vi "CRYGet Window Title Message.vi"(9 "Tooltip No":i32, 10 "No":i32, 11 "Kind":string) -> (0 "Control Label Off":string[](array[string]), 1 "Control Label On":string[](array[string]), 2 "Unicode String":string, 3 "Multibyte String":string, 4 "Control Name":string[](array[string]), 6 "Tip Strip":string[](array[string]))   [LabVIEW 2013]
uses:
  CRYMainGlobal.vi
panel:
  # "Get Window Title Message."
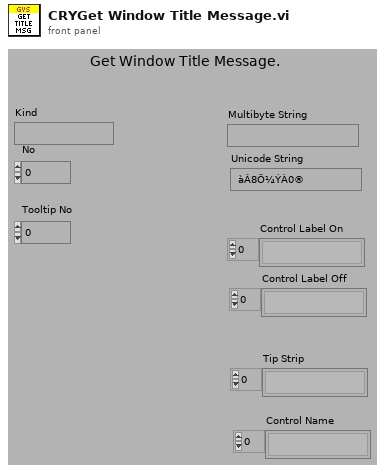
[diagram p1: front panel]
types:
  T1 = enum32{"English", "Chinese", "Korean", "Japanese", "Russian", "Chinese traditional"}
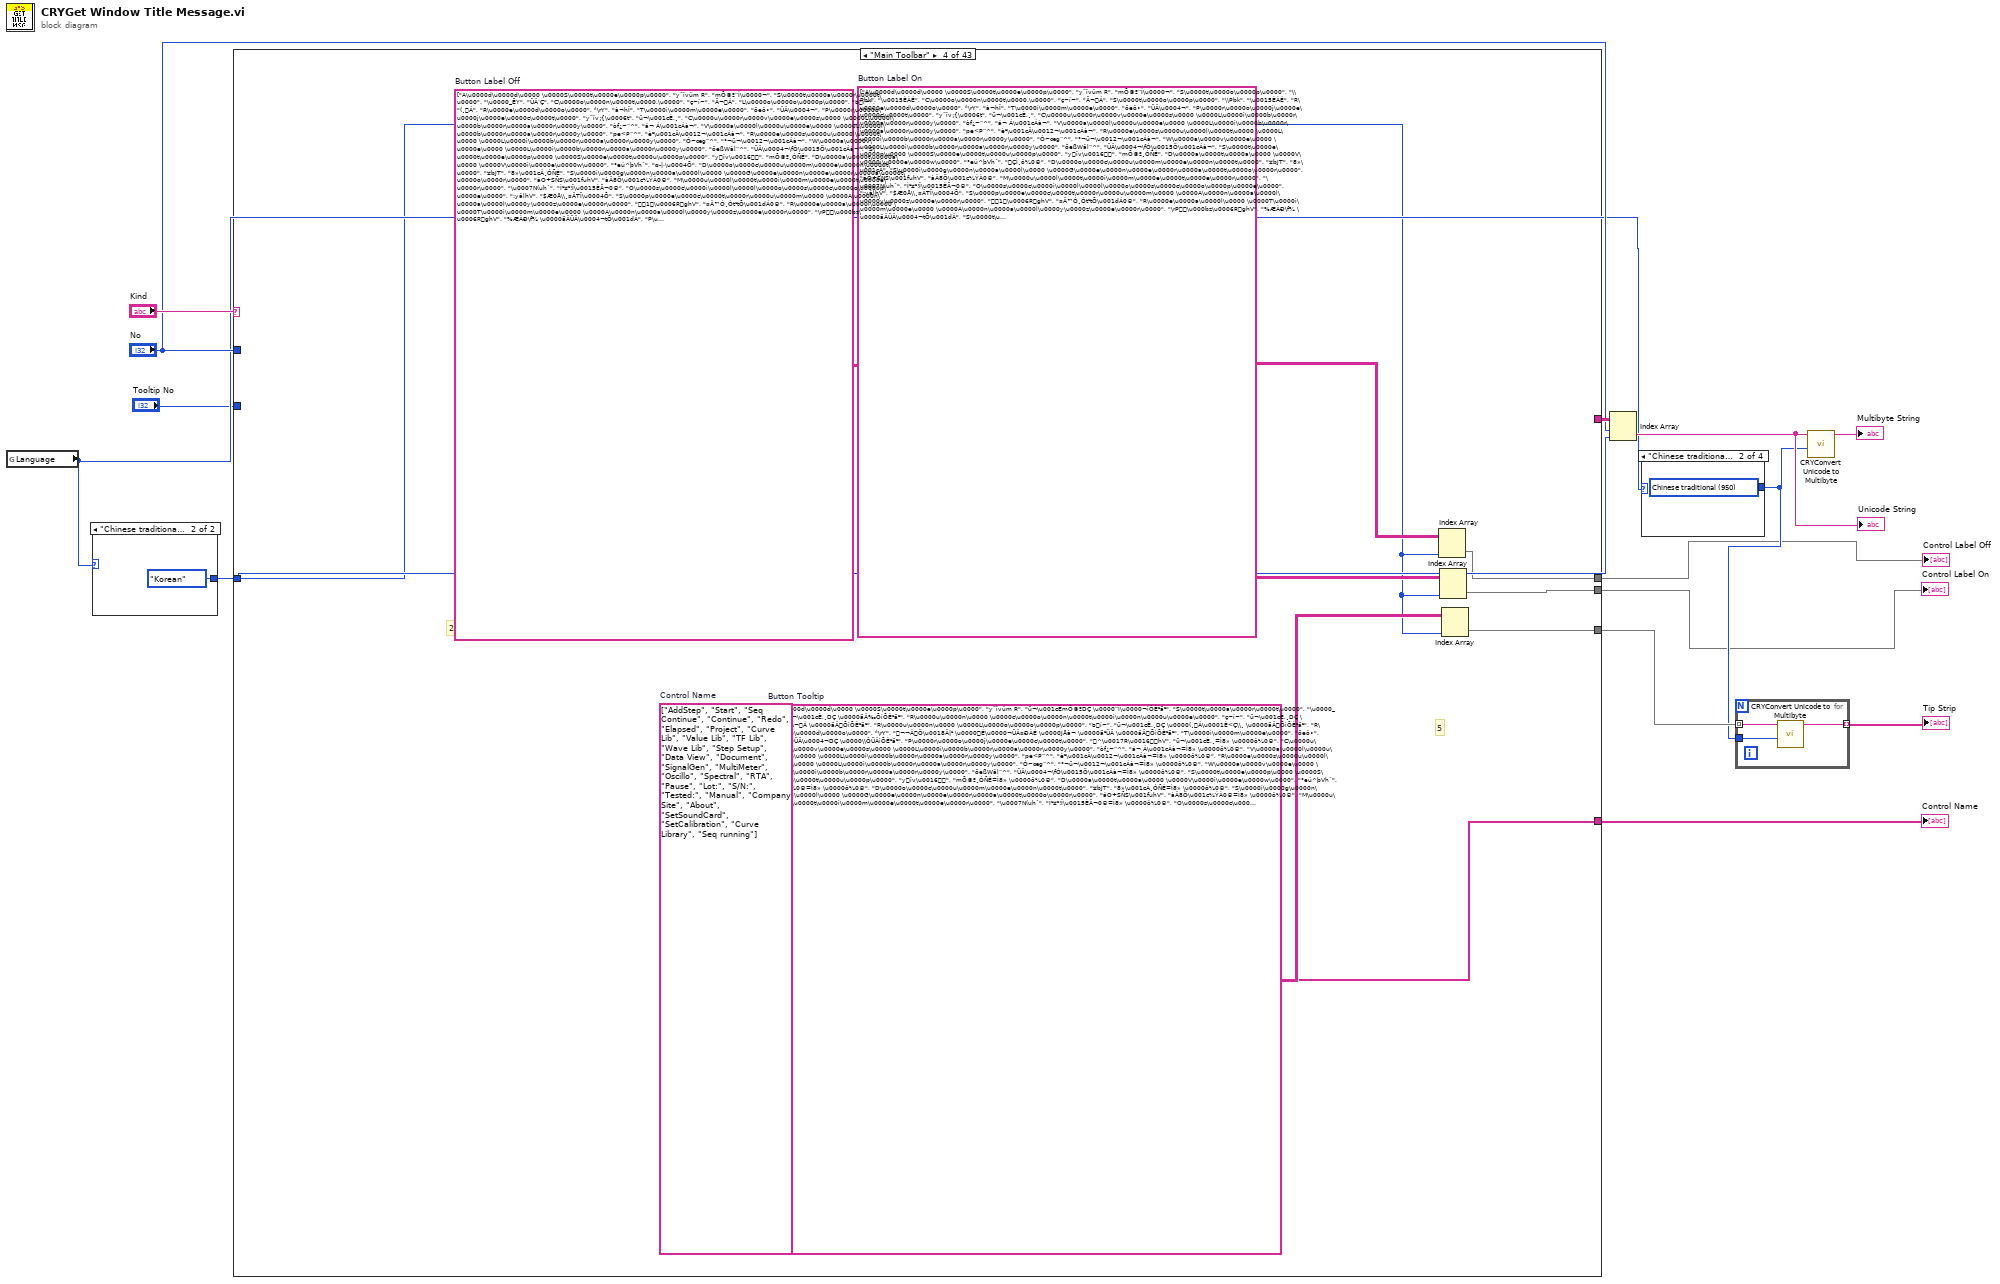
[diagram p0: block diagram]
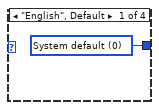
[diagram p3: hidden frame]
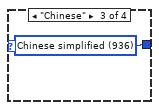
[diagram p4: hidden frame]
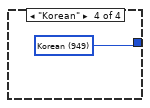
[diagram p5: hidden frame]
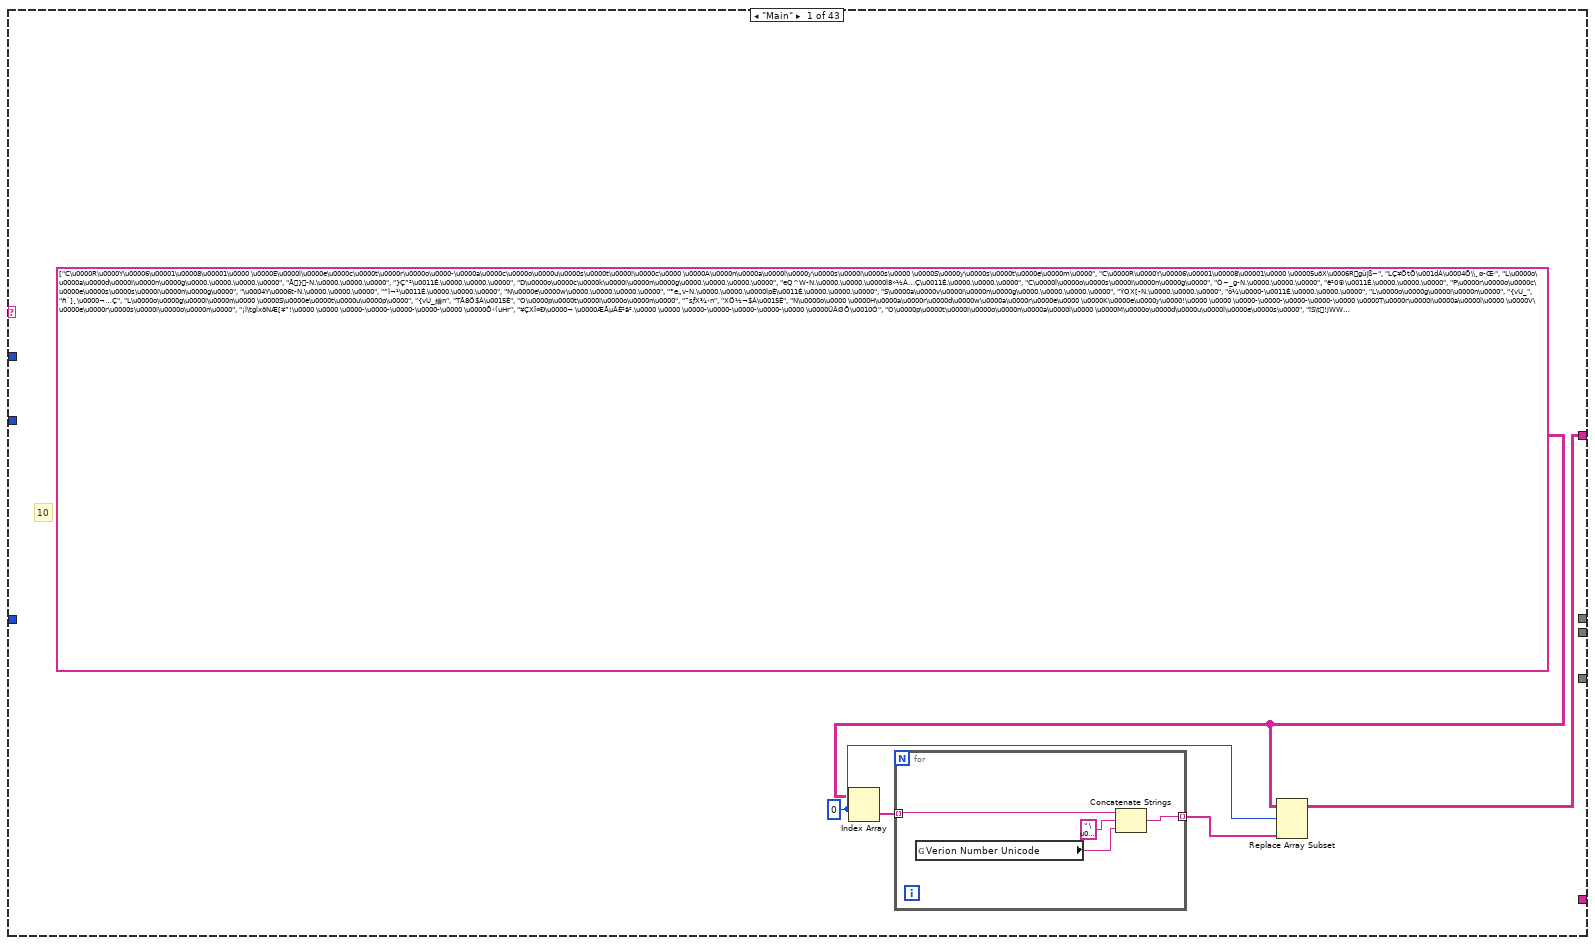
[diagram p6: hidden frame]
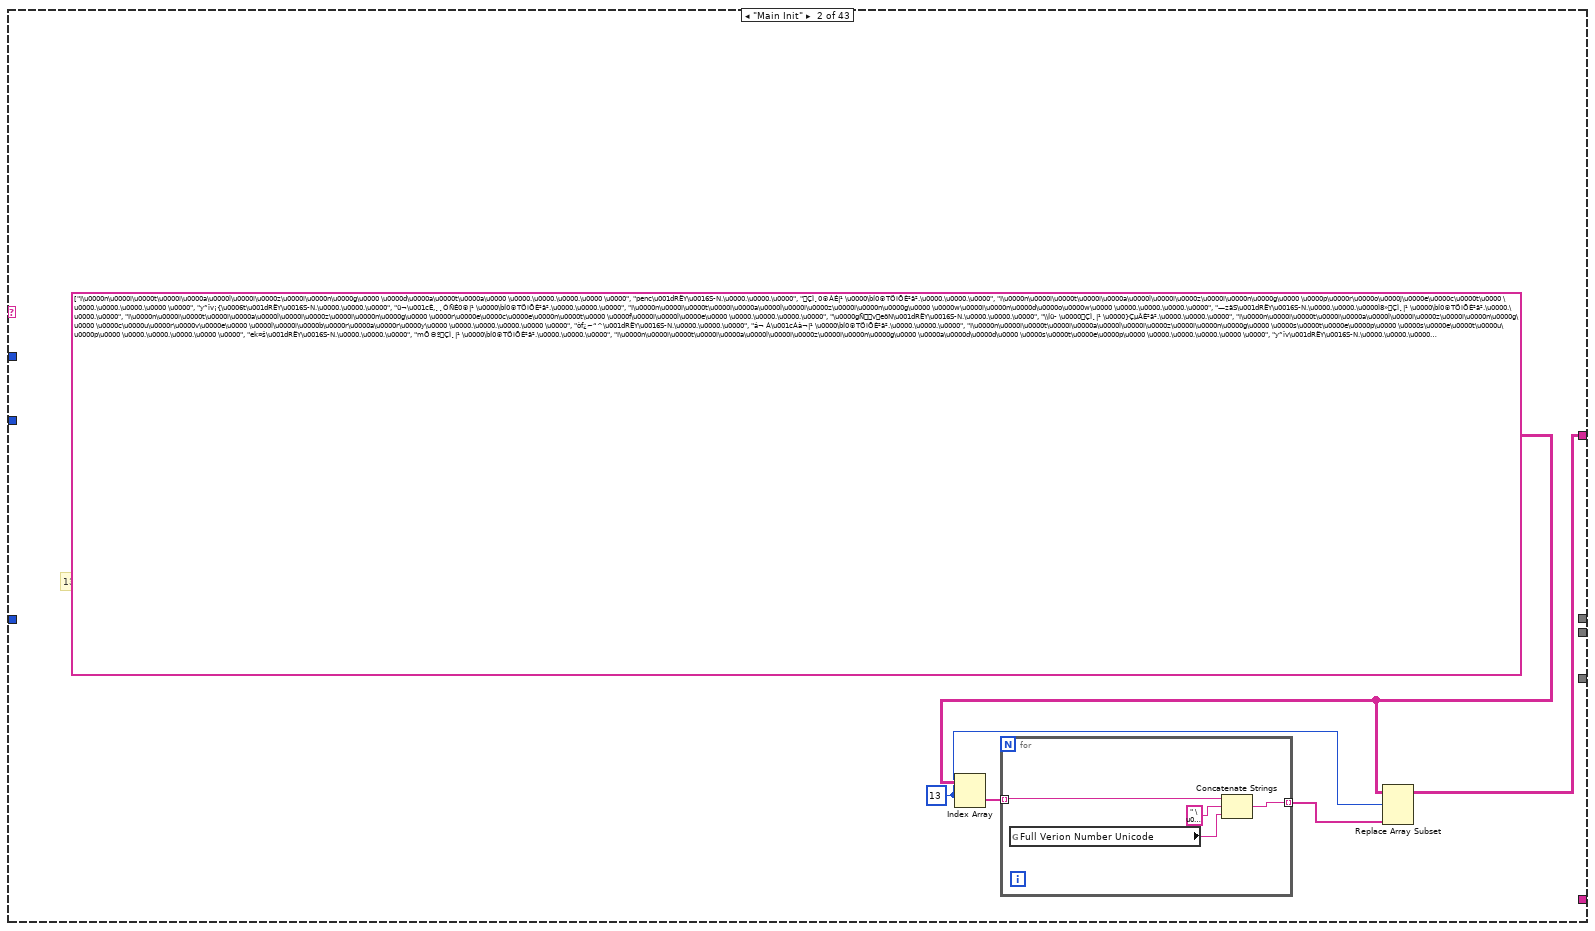
[diagram p7: hidden frame]
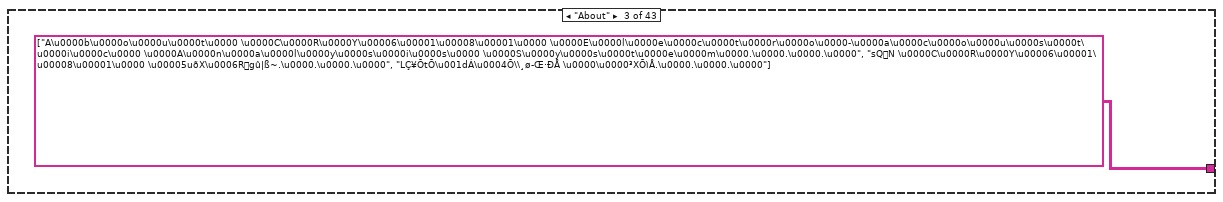
[diagram p8: hidden frame]
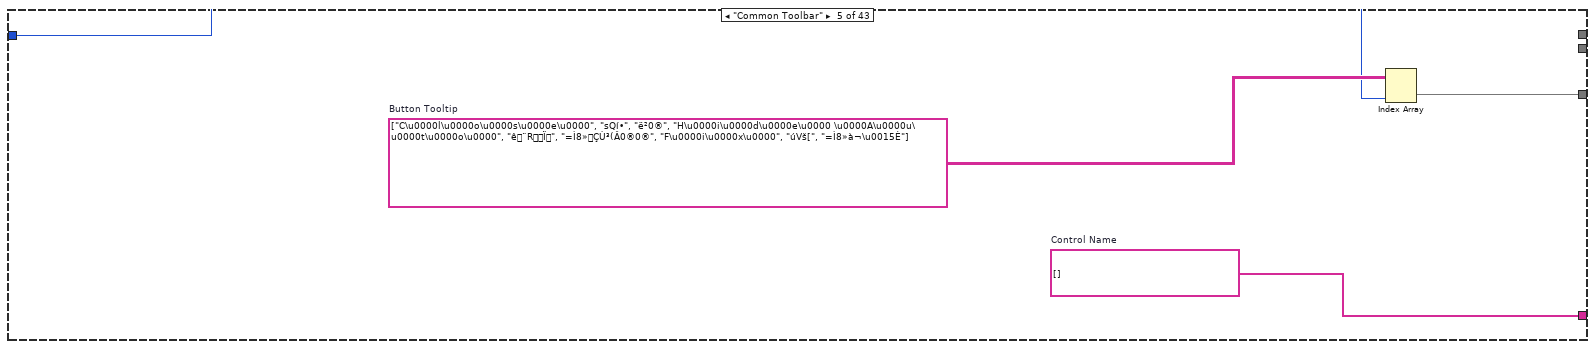
[diagram p9: hidden frame]
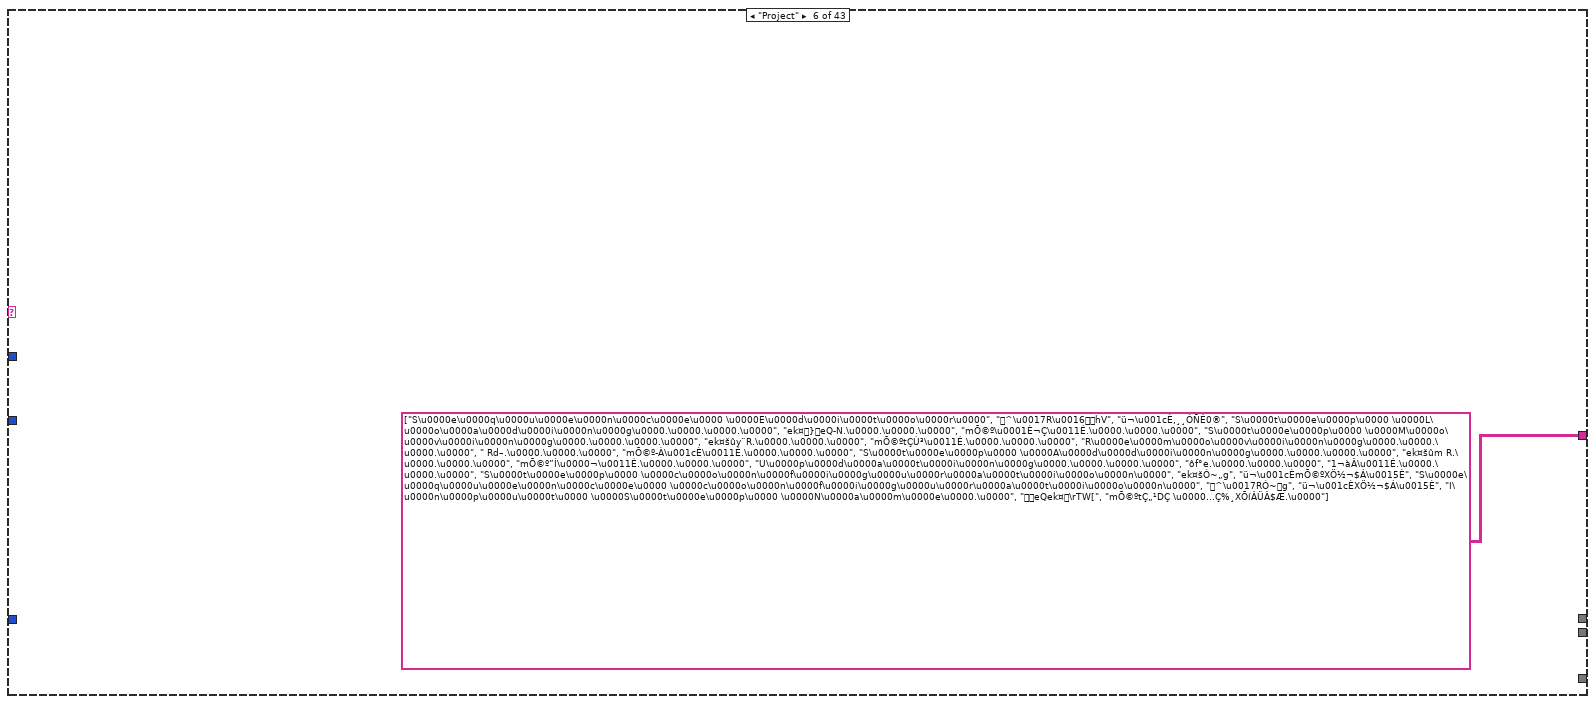
[diagram p10: hidden frame]
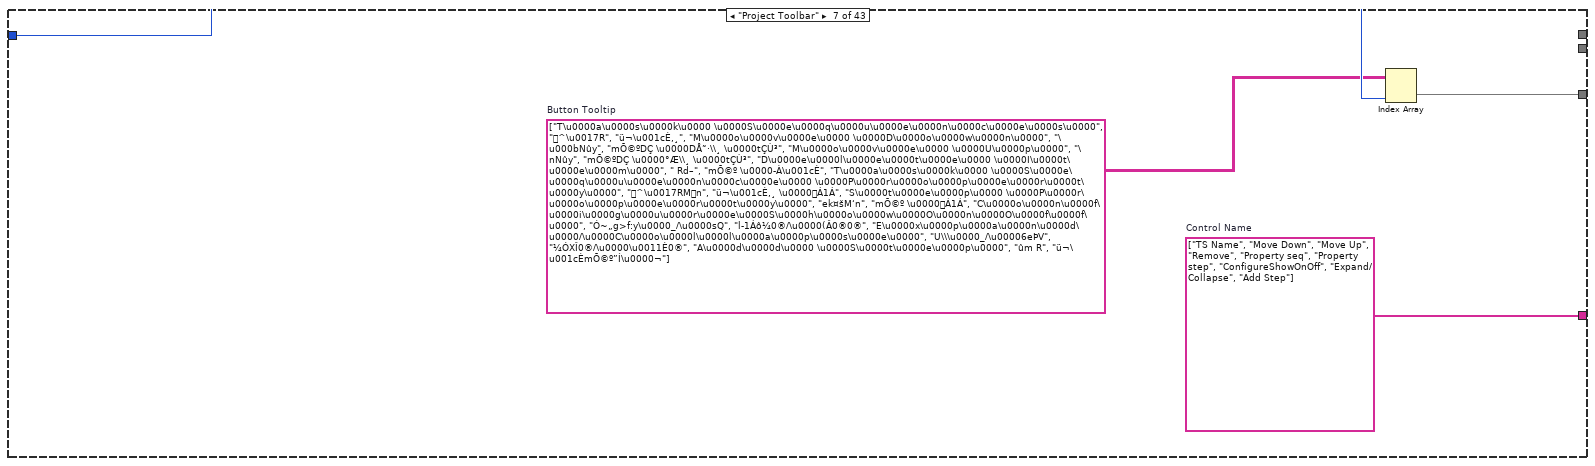
[diagram p11: hidden frame]
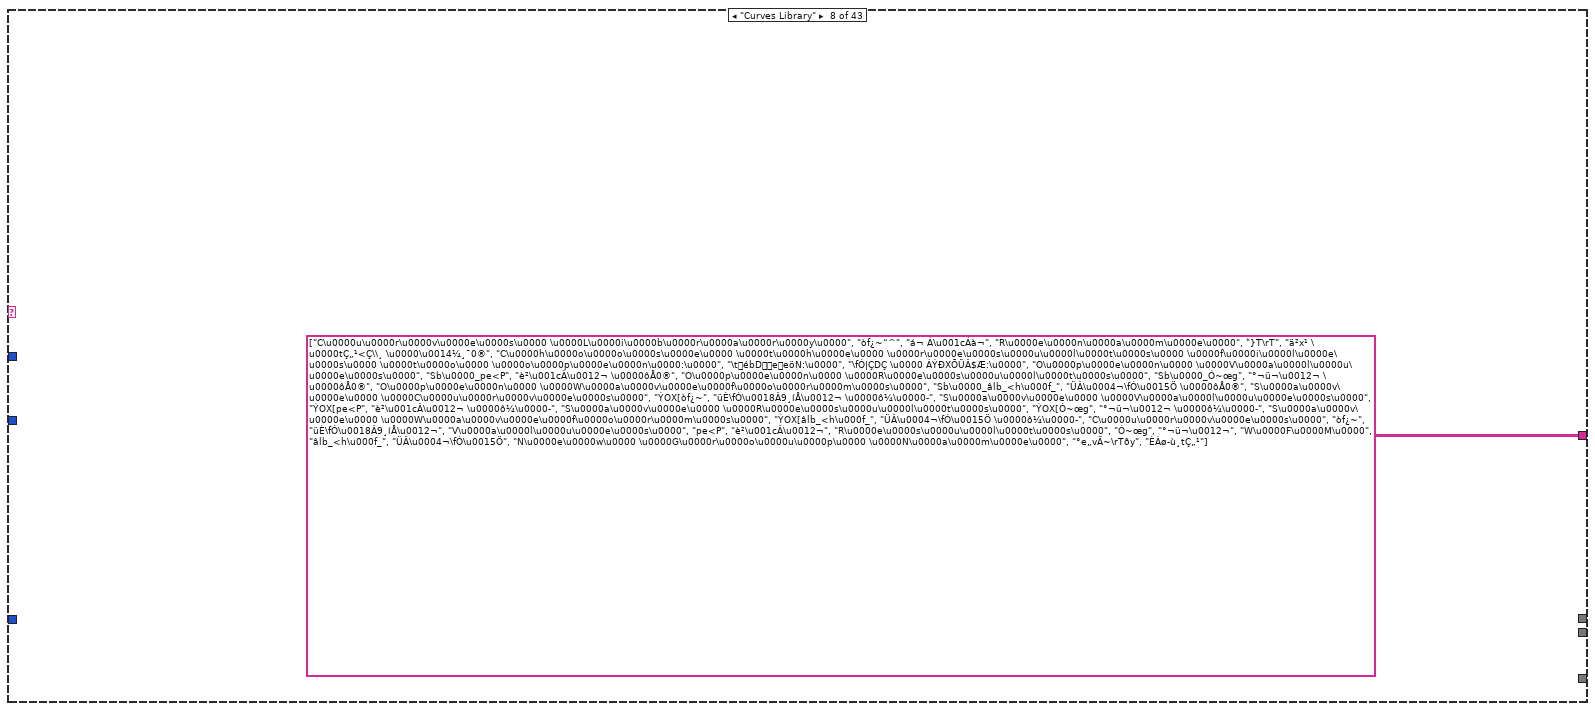
[diagram p12: hidden frame]
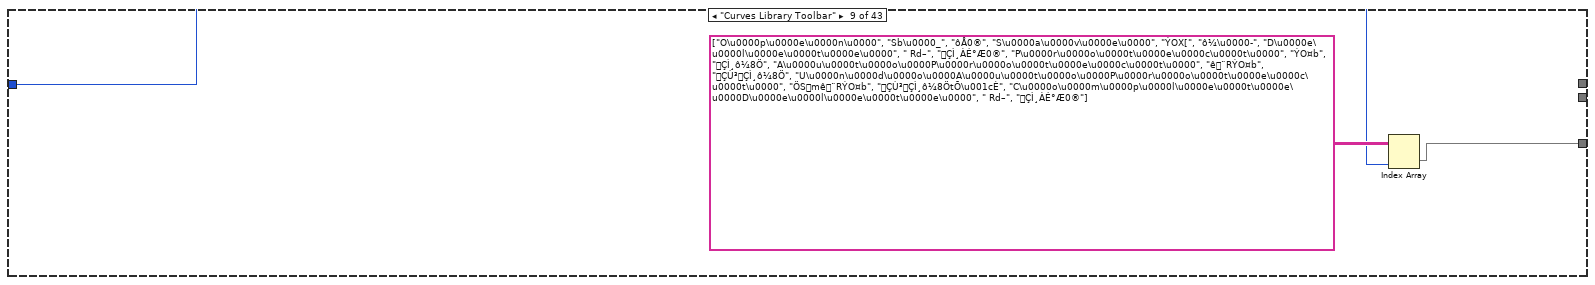
[diagram p13: hidden frame]
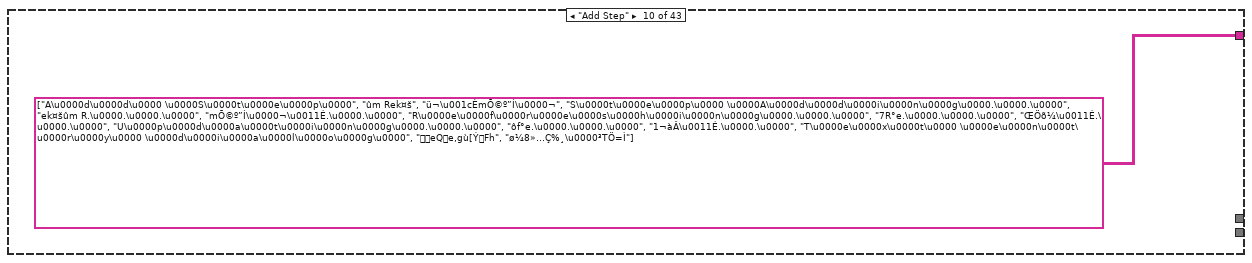
[diagram p14: hidden frame]
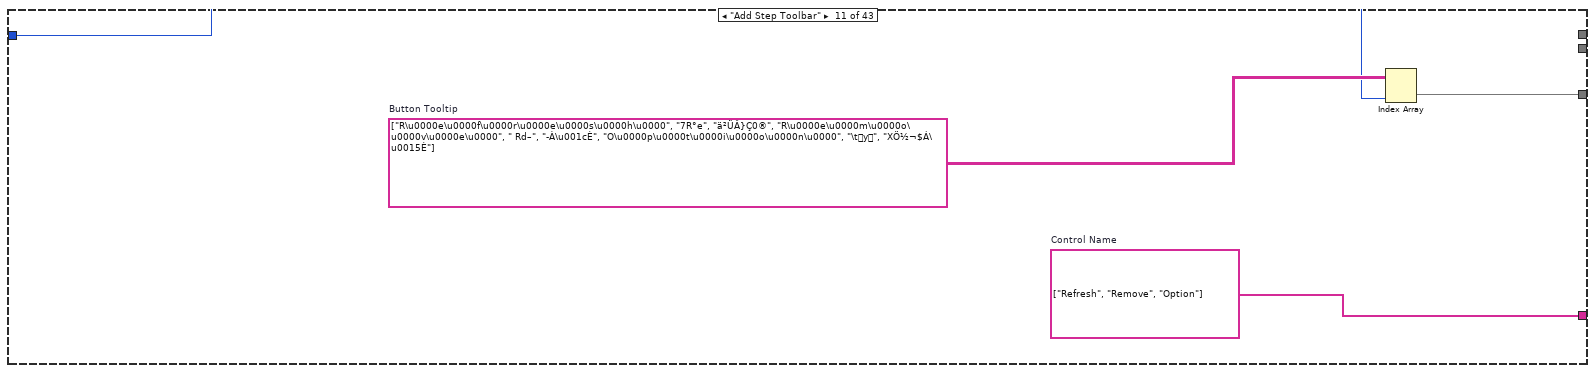
[diagram p15: hidden frame]
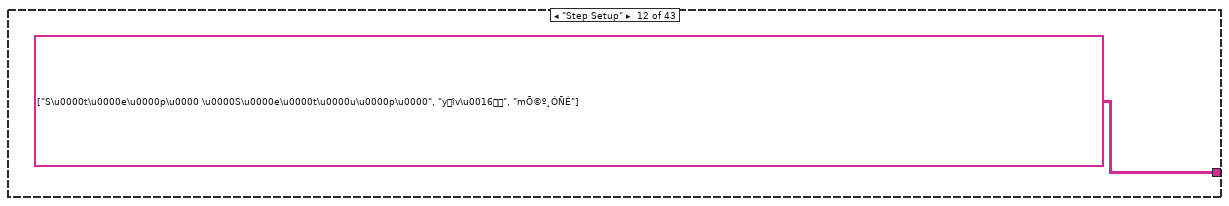
[diagram p16: hidden frame]
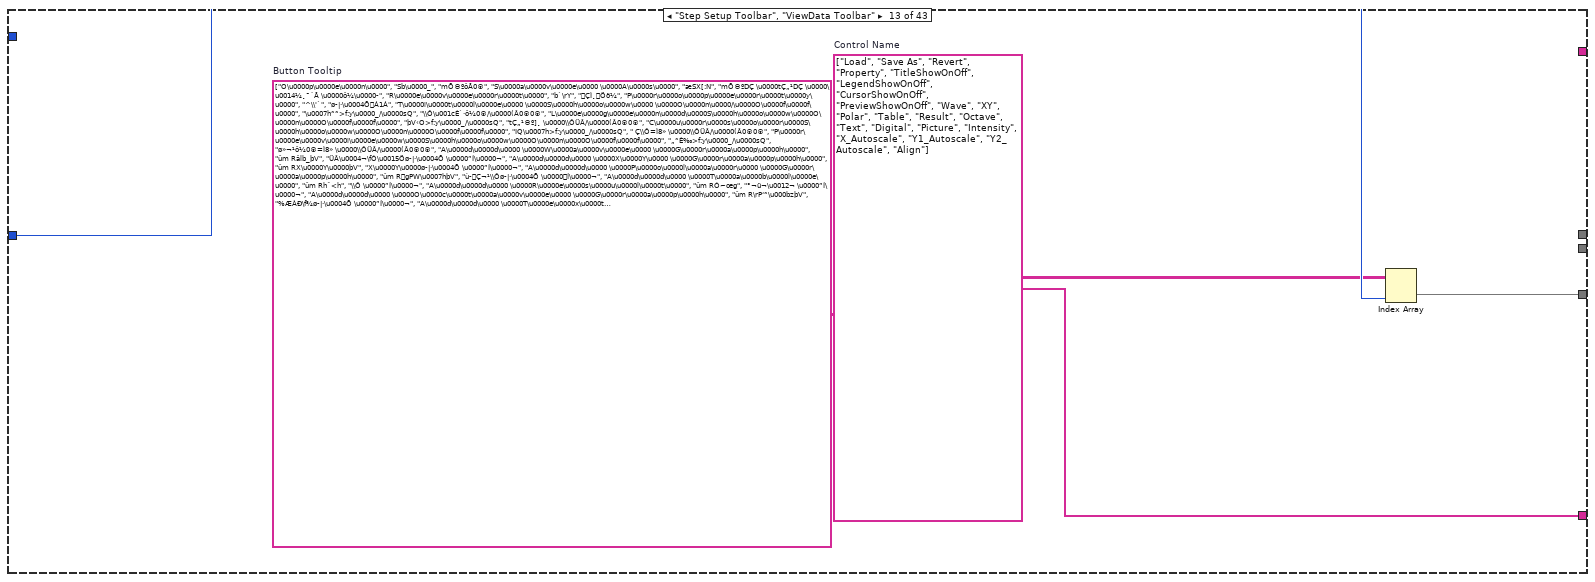
[diagram p17: hidden frame]
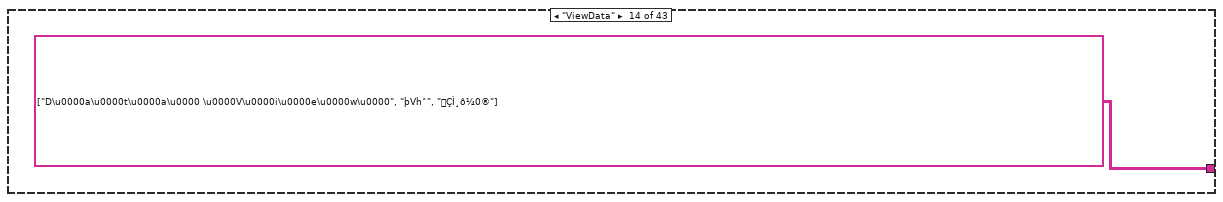
[diagram p18: hidden frame]
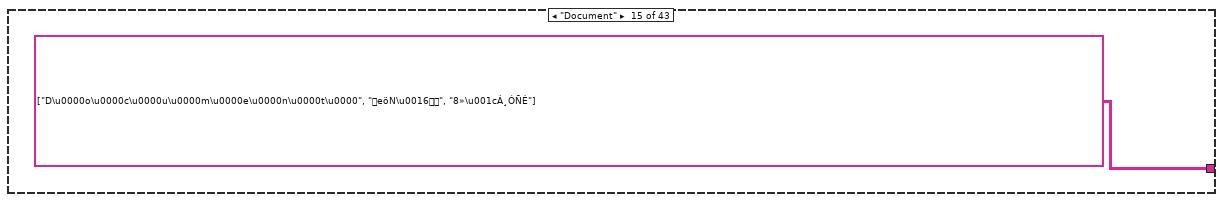
[diagram p19: hidden frame]
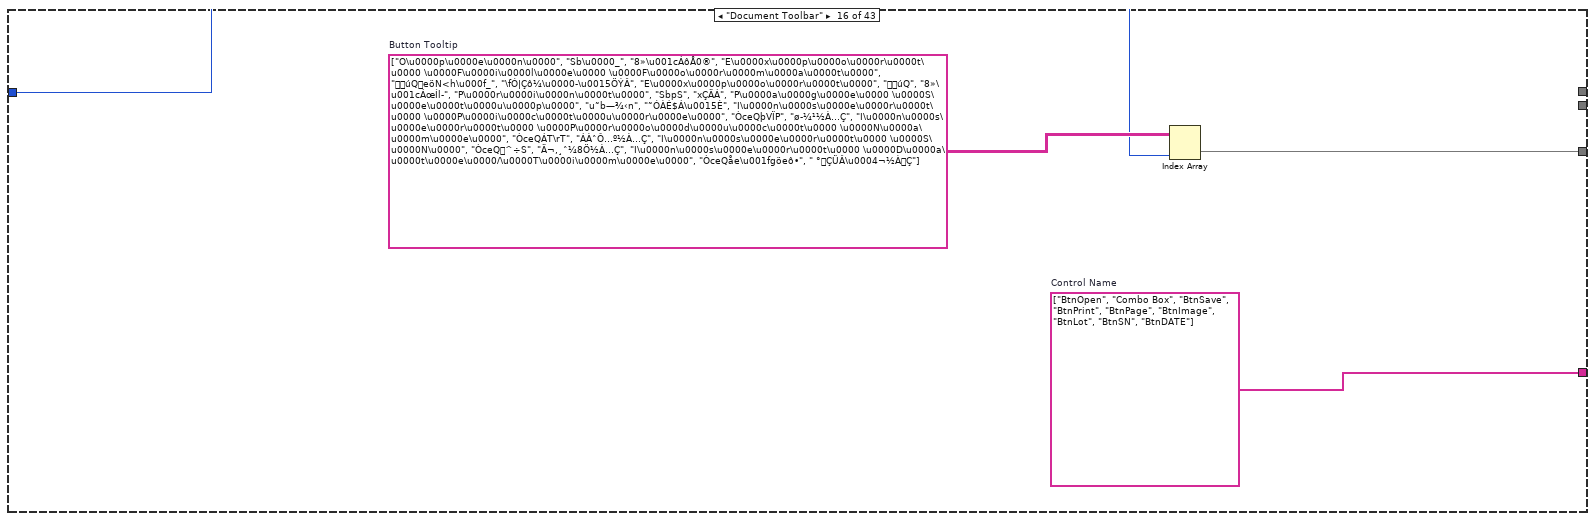
[diagram p20: hidden frame]
diagram:
  n1 = global read "CRYMainGlobal.vi" "Language"() -> (w3:T1)
  n2 = case shown="\"Chinese traditional\"" w3 {
    selector: w3 -> [w15 _]
    tunnel: [w15 T1."Korean" ("Language")] -> w2
    frame "English", Default {
    }
    frame "Chinese traditional" {
    }
  }
  n3 = case shown="\"Main Toolbar\"" "Kind" {
    tunnel: [w17 w26 string[][] [["A\u0000b\u0000o\u0000u\u0000t\u0000 \u0000C\u0000R\u0000Y\u00006\u00001\u00008\u00001\u0000 \u0000E\u0000l\u0000e\u0000c\u0000t\u0000r\u0000o\u0000-\u0000a\u0000c\u0000o\u0000u\u0000s\u0000t\u0000i\u0000c\u0000 \u0000A\u0000n\u0000a\u0000l\u0000y\u0000s\u0000i\u0000s\u0000 \u0000S\u0000y\u0000s\u0000t\u0000e\u0000m\u0000.\u0000.\u0000.\u0000", "sQN \u0000C\u0000R\u0000Y\u00006\u00001\u00008\u00001\u0000 \u00005uðX\u0006Rgû|ß~.\u0000.\u0000.\u0000", "LÇ¥ÕtÕ\u001dÁ\u0004Õ\\¸ø­Œ·ÐÅ \u0000\u0000³XÕìÅ.\u0000.\u0000.\u0000"]] _ _ string[][] [["S\u0000e\u0000q\u0000u\u0000e\u0000n\u0000c\u0000e\u0000 \u0000E\u0000d\u0000i\u0000t\u0000o\u0000r\u0000", "^\u0017R\u0016hV", "ü¬\u001cÈ,¸¸ÓÑÉ0®"], ["S\u0000t\u0000e\u0000p\u0000 \u0000L\u0000o\u0000a\u0000d\u0000i\u0000n\u0000g\u0000.\u0000.\u0000.\u0000", "ek¤}eQ-N.\u0000.\u0000.\u0000", "mÕ©º\u0001È¬Ç\u0011É.\u0000.\u0000.\u0000"], ["S\u0000t\u0000e\u0000p\u0000 \u0000M\u0000o\u0000v\u0000i\u0000n\u0000g\u0000.\u0000.\u0000.\u0000", "ek¤šûy¨R.\u0000.\u0000.\u0000", "mÕ©ºtÇÙ³\u0011É.\u0000.\u0000.\u0000"], ["R\u0000e\u0000m\u0000o\u0000v\u0000i\u0000n\u0000g\u0000.\u0000.\u0000.\u0000", " Rd–.\u0000.\u0000.\u0000", "mÕ©º­À\u001cÈ\u0011É.\u0000.\u0000.\u0000"], ["S\u0000t\u0000e\u0000p\u0000 \u0000A\u0000d\u0000d\u0000i\u0000n\u0000g\u0000.\u0000.\u0000.\u0000", "ek¤šûm R.\u0000.\u0000.\u0000", "mÕ©º”Í\u0000¬\u0011É.\u0000.\u0000.\u0000"], ["U\u0000p\u0000d\u0000a\u0000t\u0000i\u0000n\u0000g\u0000.\u0000.\u0000.\u0000", "ôf°e.\u0000.\u0000.\u0000", "1¬àÂ\u0011É.\u0000.\u0000.\u0000"], ["S\u0000t\u0000e\u0000p\u0000 \u0000c\u0000o\u0000n\u0000f\u0000i\u0000g\u0000u\u0000r\u0000a\u0000t\u0000i\u0000o\u0000n\u0000", "ek¤šÓ~„g", "ü¬\u001cÈmÕ©ºXÖ½¬$Á\u0015È"], ["S\u0000e\u0000q\u0000u\u0000e\u0000n\u0000c\u0000e\u0000 \u0000c\u0000o\u0000n\u0000f\u0000i\u0000g\u0000u\u0000r\u0000a\u0000t\u0000i\u0000o\u0000n\u0000", "^\u0017RÓ~g", "ü¬\u001cÈXÖ½¬$Á\u0015È"], ["I\u0000n\u0000p\u0000u\u0000t\u0000 \u0000S\u0000t\u0000e\u0000p\u0000 \u0000N\u0000a\u0000m\u0000e\u0000.\u0000", "eQek¤\rTW[", "mÕ©ºtÇ„¹DÇ \u0000…Ç%¸XÕíÂÜÂ$Æ.\u0000"]] _ string[][] [["C\u0000u\u0000r\u0000v\u0000e\u0000s\u0000 \u0000L\u0000i\u0000b\u0000r\u0000a\u0000r\u0000y\u0000", "òf¿~“^", "á¬ Á\u001cÁà¬"], ["R\u0000e\u0000n\u0000a\u0000m\u0000e\u0000", "͑}T\rT", "ä²x¹ \u0000tÇ„¹<Ç\\¸ \u0000\u0014¼¸¯0®"], ["C\u0000h\u0000o\u0000o\u0000s\u0000e\u0000 \u0000t\u0000h\u0000e\u0000 \u0000r\u0000e\u0000s\u0000u\u0000l\u0000t\u0000s\u0000 \u0000f\u0000i\u0000l\u0000e\u0000s\u0000 \u0000t\u0000o\u0000 \u0000o\u0000p\u0000e\u0000n\u0000:\u0000", "\tébDeeöN:\u0000", "\fÓ|ÇDÇ \u0000 ÁÝÐXÕÜÂ$Æ:\u0000"], ["O\u0000p\u0000e\u0000n\u0000 \u0000V\u0000a\u0000l\u0000u\u0000e\u0000s\u0000", "Sb\u0000_pe<P", "è²\u001cÂ\u0012¬ \u0000ôÅ0®"], ["O\u0000p\u0000e\u0000n\u0000 \u0000R\u0000e\u0000s\u0000u\u0000l\u0000t\u0000s\u0000", "Sb\u0000_Ó~œg", "°¬ü¬\u0012¬ \u0000ôÅ0®"], ["O\u0000p\u0000e\u0000n\u0000 \u0000W\u0000a\u0000v\u0000e\u0000f\u0000o\u0000r\u0000m\u0000s\u0000", "Sb\u0000_âlb_<h\u000f_", "ÜÂ\u0004¬\fÓ\u0015Ö \u0000ôÅ0®"], ["S\u0000a\u0000v\u0000e\u0000 \u0000C\u0000u\u0000r\u0000v\u0000e\u0000s\u0000", "ÝOX[òf¿~", "üÈ\fÓ\u0018Â9¸íÅ\u0012¬ \u0000ô¼\u0000­"], ["S\u0000a\u0000v\u0000e\u0000 \u0000V\u0000a\u0000l\u0000u\u0000e\u0000s\u0000", "ÝOX[pe<P", "è²\u001cÂ\u0012¬ \u0000ô¼\u0000­"], ["S\u0000a\u0000v\u0000e\u0000 \u0000R\u0000e\u0000s\u0000u\u0000l\u0000t\u0000s\u0000", "ÝOX[Ó~œg", "°¬ü¬\u0012¬ \u0000ô¼\u0000­"], ["S\u0000a\u0000v\u0000e\u0000 \u0000W\u0000a\u0000v\u0000e\u0000f\u0000o\u0000r\u0000m\u0000s\u0000", "ÝOX[âlb_<h\u000f_", "ÜÂ\u0004¬\fÓ\u0015Ö \u0000ô¼\u0000­"], ["C\u0000u\u0000r\u0000v\u0000e\u0000s\u0000", "òf¿~", "üÈ\fÓ\u0018Â9¸íÅ\u0012¬"], ["V\u0000a\u0000l\u0000u\u0000e\u0000s\u0000", "pe<P", "è²\u001cÂ\u0012¬"], ["R\u0000e\u0000s\u0000u\u0000l\u0000t\u0000s\u0000", "Ó~œg", "°¬ü¬\u0012¬"], ["W\u0000F\u0000M\u0000", "âlb_<h\u000f_", "ÜÂ\u0004¬\fÓ\u0015Ö"], ["N\u0000e\u0000w\u0000 \u0000G\u0000r\u0000o\u0000u\u0000p\u0000 \u0000N\u0000a\u0000m\u0000e\u0000", "°e„vÄ~\rTðy", "ÈÀø­ù¸tÇ„¹"]] _ string[][] [["A\u0000d\u0000d\u0000 \u0000S\u0000t\u0000e\u0000p\u0000", "ûm Rek¤š", "ü¬\u001cÈmÕ©º”Í\u0000¬"], ["S\u0000t\u0000e\u0000p\u0000 \u0000A\u0000d\u0000d\u0000i\u0000n\u0000g\u0000.\u0000.\u0000", "ek¤šûm R.\u0000.\u0000.\u0000", "mÕ©º”Í\u0000¬\u0011É.\u0000.\u0000"], ["R\u0000e\u0000f\u0000r\u0000e\u0000s\u0000h\u0000i\u0000n\u0000g\u0000.\u0000.\u0000", "7R°e.\u0000.\u0000.\u0000", "ŒÖõ¼\u0011É.\u0000.\u0000"], ["U\u0000p\u0000d\u0000a\u0000t\u0000i\u0000n\u0000g\u0000.\u0000.\u0000", "ôf°e.\u0000.\u0000.\u0000", "1¬àÂ\u0011É.\u0000.\u0000"], ["T\u0000e\u0000x\u0000t\u0000 \u0000e\u0000n\u0000t\u0000r\u0000y\u0000 \u0000d\u0000i\u0000a\u0000l\u0000o\u0000g\u0000", "eQe,gù[ÝFh", "ø¼8»…Ç%¸\u0000³TÖ=Ì"]] _ string[][] [["S\u0000t\u0000e\u0000p\u0000 \u0000S\u0000e\u0000t\u0000u\u0000p\u0000", "yîv\u0016", "mÕ©º¸ÓÑÉ"]] _ string[][] [["D\u0000a\u0000t\u0000a\u0000 \u0000V\u0000i\u0000e\u0000w\u0000", "þVhˆ", "ÇÌ¸ô¼0®"]] string[][] [["D\u0000o\u0000c\u0000u\u0000m\u0000e\u0000n\u0000t\u0000", "eöN\u0016", "8»\u001cÁ¸ÓÑÉ"]] _ string[][] [["R\u0000u\u0000n\u0000 \u0000P\u0000r\u0000o\u0000j\u0000e\u0000c\u0000t\u0000", "yîvÐL", "ü¬\u001cÈ,¸ \u0000äÂ‰Õ"]] string[][] [["W\u0000a\u0000v\u0000e\u0000 \u0000G\u0000r\u0000a\u0000p\u0000h\u0000", "âlþVhˆ", "ÜÂ\u0004¬\fÓ\u0015Öø­|·\u0004Õ"], ["W\u0000a\u0000v\u0000e\u0000 \u0000G\u0000r\u0000a\u0000p\u0000h\u0000 \u0000P\u0000r\u0000o\u0000p\u0000e\u0000r\u0000t\u0000y\u0000", "âlþVhˆ^\\'`", "ÜÂ\u0004¬\fÓ\u0015Öø­|·\u0004ÕÁ1Á"]] string[][] [["X\u0000Y\u0000 \u0000G\u0000r\u0000a\u0000p\u0000h\u0000", "X\u0000Y\u0000þVhˆ", "X\u0000Y\u0000ø­|·\u0004Õ"], ["X\u0000Y\u0000 \u0000G\u0000r\u0000a\u0000p\u0000h\u0000 \u0000P\u0000r\u0000o\u0000p\u0000e\u0000r\u0000t\u0000y\u0000", "X\u0000Y\u0000þVhˆ^\\'`", "X\u0000Y\u0000ø­|·\u0004ÕÁ1Á"]] string[][] [["D\u0000i\u0000g\u0000i\u0000t\u0000a\u0000l\u0000 \u0000G\u0000r\u0000a\u0000p\u0000h\u0000", "peW[þVhˆ", "\u0018ÂÇàÂ8Öø­|·\u0004Õ"], ["D\u0000i\u0000g\u0000i\u0000t\u0000a\u0000l\u0000 \u0000G\u0000r\u0000a\u0000p\u0000h\u0000 \u0000P\u0000r\u0000o\u0000p\u0000e\u0000r\u0000t\u0000y\u0000", "peW[þVhˆ^\\'`", "\u0018ÂÇàÂ8Öø­|·\u0004ÕÁ1Á"]] string[][] [["O\u0000c\u0000t\u0000a\u0000v\u0000e\u0000 \u0000G\u0000r\u0000a\u0000p\u0000h\u0000", "\rP‘˜\u000bzþVhˆ", "%ÆÀÐ\f¾ø­|·\u0004Õ"], ["O\u0000c\u0000t\u0000a\u0000v\u0000e\u0000 \u0000G\u0000r\u0000a\u0000p\u0000h\u0000 \u0000P\u0000r\u0000o\u0000p\u0000e\u0000r\u0000t\u0000y\u0000", "\rP‘˜\u000bzþVhˆ^\\'`", "%ÆÀÐ\f¾ø­|·\u0004ÕÁ1Á"]] string[][] [["P\u0000o\u0000l\u0000a\u0000r\u0000 \u0000G\u0000r\u0000a\u0000p\u0000h\u0000", "gPW\u0007hþVh", "ù­Ç¬¹\\Ôø­|·\u0004Õ"], ["P\u0000o\u0000l\u0000a\u0000r\u0000 \u0000G\u0000r\u0000a\u0000p\u0000h\u0000 \u0000P\u0000r\u0000o\u0000p\u0000e\u0000r\u0000t\u0000y\u0000 \u0000", "gPW\u0007hþVh^\\'`", "ù­Ç¬¹\\Ôø­|·\u0004ÕÁ1Á"]] string[][] [["T\u0000e\u0000x\u0000t\u0000", ",g‡e", "ø¼8»"], ["T\u0000e\u0000x\u0000t\u0000 \u0000P\u0000r\u0000o\u0000p\u0000e\u0000r\u0000t\u0000y\u0000", ",g‡e^\\'`", "ø¼8»Á1Á"]] string[][] [["T\u0000a\u0000b\u0000l\u0000e\u0000 \u0000G\u0000r\u0000a\u0000p\u0000h\u0000", "hˆ", "\\Ô"], ["T\u0000a\u0000b\u0000l\u0000e\u0000 \u0000G\u0000r\u0000a\u0000p\u0000h\u0000 \u0000P\u0000r\u0000o\u0000p\u0000e\u0000r\u0000t\u0000y\u0000", "hˆ^\\'`", "\\ÔÁ1Á"]] string[][] [["P\u0000i\u0000c\u0000t\u0000u\u0000r\u0000e\u0000 \u0000G\u0000r\u0000a\u0000p\u0000h\u0000", "þVÏP", "ø­¼¹"], ["P\u0000i\u0000c\u0000t\u0000u\u0000r\u0000e\u0000 \u0000G\u0000r\u0000a\u0000p\u0000h\u0000 \u0000P\u0000r\u0000o\u0000p\u0000e\u0000r\u0000t\u0000y\u0000", "þVÏP^\\'`", "ø­¼¹Á1Á"]] string[][] [["R\u0000e\u0000s\u0000u\u0000l\u0000t\u0000 \u0000G\u0000r\u0000a\u0000p\u0000h\u0000", "Ó~œg", "°¬ü¬\u0012¬"], ["R\u0000e\u0000s\u0000u\u0000l\u0000t\u0000 \u0000G\u0000r\u0000a\u0000p\u0000h\u0000 \u0000P\u0000r\u0000o\u0000p\u0000e\u0000r\u0000t\u0000y\u0000", "Ó~œg^\\'`", "°¬ü¬\u0012¬Á1Á"]] string[][] [["I\u0000n\u0000t\u0000e\u0000n\u0000s\u0000i\u0000t\u0000y\u0000 \u0000G\u0000r\u0000a\u0000p\u0000h\u0000", "Æ[¦^þVhˆ", "\u0000¼Ä³ø­|·\u0004Õ"], ["I\u0000n\u0000t\u0000e\u0000n\u0000s\u0000i\u0000t\u0000y\u0000 \u0000G\u0000r\u0000a\u0000p\u0000h\u0000 \u0000P\u0000r\u0000o\u0000p\u0000e\u0000r\u0000t\u0000y\u0000", "Æ[¦^þVhˆ^\\'`", "\u0000¼Ä³ø­|·\u0004ÕÁ1Á"]] string[][] [["S\u0000o\u0000u\u0000n\u0000d\u0000C\u0000a\u0000r\u0000d\u0000", "ðXaS", "ŒÁ¬¹tÎÜ´"]] string[][] [["C\u0000a\u0000l\u0000i\u0000b\u0000r\u0000a\u0000t\u0000i\u0000o\u0000n\u0000 \u0000P\u0000a\u0000r\u0000a\u0000m\u0000e\u0000t\u0000e\u0000r\u0000s\u0000 \u0000T\u0000a\u0000b\u0000l\u0000e\u0000", "!hÆQÂSpehˆ", "P­\u0000É\fÓ|·Tº0Ñ\\Ô"], ["M\u0000i\u0000c\u0000r\u0000o\u0000p\u0000h\u0000o\u0000n\u0000e\u0000 \u0000C\u0000a\u0000l\u0000i\u0000b\u0000r\u0000a\u0000t\u0000i\u0000o\u0000n\u0000", " OðXhV!hÆQ", "È¹tÇlÐP­\u0000É"], ["U\u0000n\u0000i\u0000t\u0000s\u0000 \u0000S\u0000e\u0000t\u0000u\u0000p\u0000", "USMO¾‹š[", "è²\u0004Ç$Á\u0015È"], ["S\u0000i\u0000g\u0000n\u0000a\u0000l\u0000 \u0000T\u0000y\u0000p\u0000e\u0000 \u0000S\u0000e\u0000l\u0000e\u0000c\u0000t\u0000i\u0000o\u0000n\u0000", "áO÷S{|W\téb", "àÂ8Ö\u0015ÖÜÐ \u0000 ÁÝÐ"], ["C\u0000a\u0000l\u0000i\u0000b\u0000r\u0000a\u0000t\u0000i\u0000o\u0000n\u0000", "!hÆQ", "P­\u0000É"]] string[][] [["T\u0000e\u0000x\u0000t\u0000 \u0000p\u0000r\u0000e\u0000f\u0000e\u0000r\u0000e\u0000n\u0000c\u0000e\u0000", "e,g\u0018O\t", "ø¼8»°Æ Á ÁÝÐ"], ["S\u0000e\u0000t\u0000t\u0000i\u0000n\u0000g\u0000 \u0000D\u0000i\u0000g\u0000i\u0000t\u0000a\u0000l\u0000 \u0000I\u0000/\u0000O\u0000", "¾npeW[eQ/\u0000úQ", "\u0018ÂÇÇÍl­$Á\u0015È"]] string[][] [["S\u0000t\u0000i\u0000m\u0000u\u0000l\u0000u\u0000s\u0000 \u0000E\u0000d\u0000i\u0000t\u0000o\u0000r\u0000", "Ào±R\u0016", "Çù­àÂ8Ö¸ÓÑÉ0®"]] string[][] [["H\u0000a\u0000r\u0000m\u0000o\u0000n\u0000i\u0000c\u0000 \u0000L\u0000i\u0000s\u0000t\u0000 \u0000E\u0000d\u0000i\u0000t\u0000o\u0000r\u0000", "\u0010âl\u0017Rh\u0016", "0¼pÈ\fÓ©º]¸ \u0000¸ÓÑÉ"]] string[][] [["S\u0000e\u0000a\u0000r\u0000c\u0000h\u0000 \u0000R\u0000a\u0000n\u0000g\u0000e\u0000 \u0000E\u0000d\u0000i\u0000t\u0000o\u0000r\u0000", "\u001cd\"}\u0003ôV\u0016", "ÐÐÉÀ”¼\u0004Ç¸ÓÑÉ"], ["U\u0000s\u0000e\u0000r\u0000 \u0000E\u0000q\u0000u\u0000a\u0000t\u0000i\u0000o\u0000n\u0000 \u0000P\u0000a\u0000r\u0000a\u0000m\u0000e\u0000t\u0000e\u0000r\u0000s\u0000 \u0000T\u0000a\u0000b\u0000l\u0000e\u0000", "(u7b¹e\u000bzÂSpehˆ", "¬À©ÆÇ)¼\u0015ÈÝÂÀ¼\u0018Â\\Ô"]] string[][] [["R\u0000e\u0000p\u0000l\u0000a\u0000c\u0000e\u0000 \u0000e\u0000x\u0000i\u0000s\u0000t\u0000i\u0000n\u0000g\u0000 \u0000F\u0000i\u0000l\u0000e\u0000?\u0000", "ÿfbcò]X[(W„v‡eöN\u0017T?\u0000", "tÇø» \u0000ˆÇ”² \u0000\fÓ|ÇDÇ \u0000P­´ÌXÕ ¬µÂÈ²L®?\u0000"], ["P\u0000l\u0000e\u0000a\u0000s\u0000e\u0000 \u0000e\u0000n\u0000t\u0000e\u0000r\u0000 \u0000a\u0000 \u0000n\u0000a\u0000m\u0000e\u0000", "÷eQ\rTW[", "tÇ„¹DÇ \u0000…Ç%¸XÕíÂÜÂ$Æ.\u0000"], ["E\u0000n\u0000t\u0000e\u0000r\u0000 \u0000c\u0000o\u0000m\u0000m\u0000e\u0000n\u0000t\u0000 \u0000f\u0000o\u0000r\u0000 \u0000d\u0000a\u0000t\u0000a\u0000f\u0000i\u0000l\u0000e\u0000:\u0000", "eQeöNèlã.\u0000", "ÇÌ¸\fÓ|ÇXÇ \u0000üÈtÕ|¹ \u0000Ç%¸XÕíÂÜÂ$Æ.\u0000"]] string[][] [["I\u0000n\u0000p\u0000u\u0000t\u0000 \u0000S\u0000e\u0000r\u0000i\u0000a\u0000l\u0000 \u0000N\u0000o\u0000", "eQ^\u0017R÷S", "Ä¬,¸ˆ¼8Ö…Ç%¸"]] string[][] [["N\u0000u\u0000m\u0000b\u0000e\u0000r\u0000 \u0000F\u0000o\u0000r\u0000m\u0000a\u0000t\u0000", "penc<h\u000f_", "\u0012¬$Á\u0015È"], ["A\u0000d\u0000d\u0000 \u0000C\u0000u\u0000r\u0000v\u0000e\u0000 \u0000N\u0000a\u0000m\u0000e\u0000", " R\nNòf¿~\rTW[", "á¬ ÁtÇ„¹¨Ì\u0000¬"], ["I\u0000m\u0000p\u0000o\u0000r\u0000t\u0000 \u0000W\u0000i\u0000z\u0000a\u0000r\u0000d\u0000 \u0000p\u00001\u0000", "ü[eQ\u0011Tü[ \u00001\u0000", "ø¼8»\fÓ|Ç\\¸€½0Ñ \u0000…Çl­-\u0000x¬LÇ \u00001\u0000"], ["I\u0000m\u0000p\u0000o\u0000r\u0000t\u0000 \u0000W\u0000i\u0000z\u0000a\u0000r\u0000d\u0000 \u0000p\u00002\u0000", "ü[eQ\u0011Tü[ \u00002\u0000", "ø¼8»\fÓ|Ç\\¸€½0Ñ \u0000…Çl­-\u0000x¬LÇ \u00002\u0000"], ["I\u0000m\u0000p\u0000o\u0000r\u0000t\u0000 \u0000W\u0000i\u0000z\u0000a\u0000r\u0000d\u0000 \u0000p\u00003\u0000", "ü[eQ\u0011Tü[ \u00003\u0000", "ø¼8»\fÓ|Ç\\¸€½0Ñ \u0000…Çl­-\u0000x¬LÇ \u00003\u0000"]] string[][] [["S\u0000i\u0000g\u0000n\u0000a\u0000l\u0000 \u0000G\u0000e\u0000n\u0000e\u0000r\u0000a\u0000t\u0000o\u0000r\u0000", "áO÷SÑS\u001fuhV", "àÂ8Ö\u001c¼ÝÀ0®"]] string[][] [["M\u0000u\u0000l\u0000t\u0000i\u0000m\u0000e\u0000t\u0000e\u0000r\u0000 \u0000", "\u0007N(uhˆ", "Ì¹¥²!Î\u0015ÈÄ¬0®"]] string[][] [["S\u0000c\u0000o\u0000p\u0000e\u0000-\u0000F\u0000F\u0000T\u0000", ":yâlhV", "$Æ0Å\\¸¤ÂTÏ\u0004Õ"], ["S\u0000c\u0000o\u0000p\u0000e\u0000-\u0000F\u0000F\u0000T\u0000", "1\u0006Rg", "¤Â™Ó¸Òt¹„½\u001dÁ"]] string[][] [[" \u0000O\u0000c\u0000t\u0000a\u0000v\u0000e\u0000 \u0000R\u0000e\u0000a\u0000l\u0000 \u0000T\u0000i\u0000m\u0000e\u0000 \u0000A\u0000n\u0000a\u0000l\u0000y\u0000z\u0000e\u0000r\u0000", "\rP\u000bz\u0006RghV", "%ÆÀÐ\f¾ \u0000äÂÜÂ\u0004¬tÕ\u001dÁ"]] string[][] [["S\u0000e\u0000l\u0000e\u0000c\u0000t\u0000 \u0000S\u0000t\u0000a\u0000r\u0000t\u0000u\u0000p\u0000 \u0000C\u0000o\u0000n\u0000f\u0000i\u0000g\u0000u\u0000r\u0000a\u0000t\u0000i\u0000o\u0000n\u0000", "\téb/T¨RMn.\u0000", "äÂÜÂ\u0004¬ü¬\u001cÈ,¸XÖ½¬"]] string[][] [["C\u0000R\u0000Y\u00006\u00001\u00008\u00001\u0000 \u0000E\u0000l\u0000e\u0000c\u0000t\u0000r\u0000o\u0000-\u0000a\u0000c\u0000o\u0000u\u0000s\u0000t\u0000i\u0000c\u0000 \u0000A\u0000n\u0000a\u0000l\u0000y\u0000s\u0000i\u0000s\u0000 \u0000S\u0000y\u0000s\u0000t\u0000e\u0000m\u0000 \u0000O\u0000n\u0000e\u0000 \u00001\u0000.\u00000\u0000", "C\u0000R\u0000Y\u00006\u00001\u00008\u00001\u0000 \u00005uðX\u0006Rgû|ß~ \u0000\u0000N \u00001\u0000.\u00000\u0000", "LÇ¥ÕtÕ\u001dÁ\u0004Õ\\¸ø­Œ· \u0000XÕ˜° \u00001\u0000.\u00000\u0000"], ["C\u0000R\u0000Y\u00006\u00001\u00008\u00001\u0000 \u0000O\u0000n\u0000e\u0000-\u0000Q\u0000u\u0000c\u0000i\u0000k\u0000 \u0000L\u0000a\u0000u\u0000n\u0000c\u0000h\u0000 \u0000M\u0000e\u0000n\u0000u\u0000", "C\u0000R\u0000Y\u00006\u00001\u00008\u00001\u0000 \u00005uðX\u0006Rgû|ß~\u0000NeQOO/T¨RÜUS", "LÇ¥ÕtÕ\u001dÁ\u0004Õ\\¸ø­Œ·-\u0000`¾x¹ \u00000®Ù³ \u0000HÅ´°"]] string[][] [[""]]] -> w13
    tunnel: w2 -> [_ _ _ w37 w45 _ w52 _ w54 _ w59 _ w66 _ _ w70 _ _ _ _ _ _ _ _ _ _ _ _ _ _ _ _ _ _ _ _ _ _ _ _ _ _ _]
    tunnel: "No" -> [_ _ _ _ _ _ _ _ _ _ _ _ _ _ _ _ _ _ _ _ _ _ _ _ _ _ _ _ _ _ _ _ _ _ _ _ _ _ _ _ _ _ _]
    tunnel: [_ _ _ w42 _ _ _ _ _ _ _ _ _ _ _ _ _ _ _ _ _ _ _ _ _ _ _ _ _ _ _ _ _ _ _ _ _ _ _ _ _ _ _] -> w4
    tunnel: [_ _ _ w41 w44 _ w51 _ w55 _ w58 _ w65 _ _ w69 _ _ _ _ _ _ _ _ _ _ _ _ _ _ _ _ _ _ _ _ _ _ _ _ _ _ _] -> w8
    tunnel: [_ _ _ w40 w46 _ w49 _ _ _ w60 _ w64 _ _ w71 _ _ _ _ _ _ _ _ _ _ _ _ _ _ _ _ _ _ _ _ _ _ _ _ _ _ _] -> w9
    tunnel: [_ _ _ w36 _ _ _ _ _ _ _ _ _ _ _ _ _ _ _ _ _ _ _ _ _ _ _ _ _ _ _ _ _ _ _ _ _ _ _ _ _ _ _] -> w5
    tunnel: "Tooltip No" -> [_ _ _ _ _ _ _ _ _ _ _ _ _ _ _ _ _ _ _ _ _ _ _ _ _ _ _ _ _ _ _ _ _ _ _ _ _ _ _ _ _ _ _]
    frame "Main" {
      w20 = 0 ("disabled index (col)")
      w18 = string[][] [["C\u0000R\u0000Y\u00006\u00001\u00008\u00001\u0000 \u0000E\u0000l\u0000e\u0000c\u0000t\u0000r\u0000o\u0000-\u0000a\u0000c\u0000o\u0000u\u0000s\u0000t\u0000i\u0000c\u0000 \u0000A\u0000n\u0000a\u0000l\u0000y\u0000s\u0000i\u0000s\u0000 \u0000S\u0000y\u0000s\u0000t\u0000e\u0000m\u0000", "C\u0000R\u0000Y\u00006\u00001\u00008\u00001\u0000 \u00005uðX\u0006Rgû|ß~", "LÇ¥ÕtÕ\u001dÁ\u0004Õ\\¸ø­Œ·"], ["L\u0000o\u0000a\u0000d\u0000i\u0000n\u0000g\u0000.\u0000.\u0000.\u0000", "Å}-N.\u0000.\u0000.\u0000", "}Ç”²\u0011É.\u0000.\u0000.\u0000"], ["D\u0000o\u0000c\u0000k\u0000i\u0000n\u0000g\u0000.\u0000.\u0000.\u0000", "eQ^W-N.\u0000.\u0000.\u0000", "=Ì8»½À…Ç\u0011É.\u0000.\u0000.\u0000"], ["C\u0000l\u0000o\u0000s\u0000i\u0000n\u0000g\u0000", "Ó~_g-N.\u0000.\u0000.\u0000", "ë²0®\u0011É.\u0000.\u0000.\u0000"], ["P\u0000r\u0000o\u0000c\u0000e\u0000s\u0000s\u0000i\u0000n\u0000g\u0000", "\u0004Y\u0006t-N.\u0000.\u0000.\u0000", "˜Ì¬¹\u0011É.\u0000.\u0000.\u0000"], ["N\u0000e\u0000w\u0000.\u0000.\u0000.\u0000", "°e„v-N.\u0000.\u0000.\u0000", "=ÌpÈ\u0011É.\u0000.\u0000.\u0000"], ["S\u0000a\u0000v\u0000i\u0000n\u0000g\u0000.\u0000.\u0000.\u0000", "ÝOX[-N.\u0000.\u0000.\u0000", "ô¼\u0000­\u0011É.\u0000.\u0000.\u0000"], ["L\u0000o\u0000g\u0000i\u0000n\u0000", "{vU_", "ñ´]¸\u0000¬…Ç"], ["L\u0000o\u0000g\u0000i\u0000n\u0000 \u0000S\u0000e\u0000t\u0000u\u0000p\u0000", "{vU_緥n", "TÅ8Ö$Á\u0015È"], ["O\u0000p\u0000t\u0000i\u0000o\u0000n\u0000", "¯sƒX¾‹n", "XÖ½¬$Á\u0015È"], ["N\u0000o\u0000 \u0000H\u0000a\u0000r\u0000d\u0000w\u0000a\u0000r\u0000e\u0000 \u0000K\u0000e\u0000y\u0000!\u0000 \u0000 \u0000-\u0000-\u0000-\u0000-\u0000 \u0000T\u0000r\u0000i\u0000a\u0000l\u0000 \u0000V\u0000e\u0000r\u0000s\u0000i\u0000o\u0000n\u0000", "¡l\tglxöNÆ[¥”!\u0000 \u0000 \u0000-\u0000-\u0000-\u0000-\u0000 \u0000Õ‹(uHr", "¥ÇXÎ¤Ð\u0000¬ \u0000ÆÅµÂÈ²ä².\u0000 \u0000 \u0000-\u0000-\u0000-\u0000-\u0000 \u0000ÜÂØÕ\u0010Ó"], ["O\u0000p\u0000t\u0000i\u0000o\u0000n\u0000a\u0000l\u0000 \u0000M\u0000o\u0000d\u0000u\u0000l\u0000e\u0000s\u0000", "ïS\t!jWW", "$ÁXÎ\u001c´ \u0000¨ºÈ´ä´"]]
      # "10"
      n4 = Index Array(array=w18, index (row)=w20) -> (element=w21:string[])  [unwired: 1 in]
      n5 = for {
        tunnel: w21 -> [w25] mode=indexing
        tunnel: [w24] -> w19 mode=indexing
        n6 = global read "CRYMainGlobal.vi" "Verion Number Unicode"() -> (w23:string)
        n7 = Concatenate Strings(w25, " \u0000" ("message"), w23) -> (w24:string)
      }
      n8 = Replace Array Subset(array=w18, new element=w19, index (row)=w20) -> (w17:string[][])  [unwired: 1 in]
    }
    frame "Main Init" {
      w28 = 13 ("disabled index (col)")
      w29 = string[][] [["I\u0000n\u0000i\u0000t\u0000i\u0000a\u0000l\u0000i\u0000z\u0000i\u0000n\u0000g\u0000 \u0000d\u0000a\u0000t\u0000a\u0000 \u0000.\u0000.\u0000.\u0000 \u0000", "penc\u001dRËY\u0016S-N.\u0000.\u0000.\u0000", "ÇÌ¸0®ÀÉ|¹ \u0000\bÍ0®TÖiÕÈ²ä².\u0000.\u0000.\u0000"], ["I\u0000n\u0000i\u0000t\u0000i\u0000a\u0000l\u0000i\u0000z\u0000i\u0000n\u0000g\u0000 \u0000p\u0000r\u0000o\u0000j\u0000e\u0000c\u0000t\u0000 \u0000.\u0000.\u0000.\u0000 \u0000", "y˜îv¡{\u0006t\u001dRËY\u0016S-N.\u0000.\u0000.\u0000", "ü¬\u001cÈ,¸¸ÓÑÉ0®|¹ \u0000\bÍ0®TÖiÕÈ²ä².\u0000.\u0000.\u0000"], ["I\u0000n\u0000i\u0000t\u0000i\u0000a\u0000l\u0000i\u0000z\u0000i\u0000n\u0000g\u0000 \u0000w\u0000i\u0000n\u0000d\u0000o\u0000w\u0000 \u0000.\u0000.\u0000.\u0000", "—zãS\u001dRËY\u0016S-N.\u0000.\u0000.\u0000", "=Ì8»ÇÌ¸|¹ \u0000\bÍ0®TÖiÕÈ²ä².\u0000.\u0000.\u0000"], ["I\u0000n\u0000i\u0000t\u0000i\u0000a\u0000l\u0000i\u0000z\u0000i\u0000n\u0000g\u0000 \u0000r\u0000e\u0000c\u0000e\u0000n\u0000t\u0000 \u0000f\u0000i\u0000l\u0000e\u0000 \u0000.\u0000.\u0000.\u0000", "\u0000gÑveöN\u001dRËY\u0016S-N.\u0000.\u0000.\u0000", "\\Íü­ \u0000ÇÌ¸|¹ \u0000}ÇµÂÈ²ä².\u0000.\u0000.\u0000"], ["I\u0000n\u0000i\u0000t\u0000i\u0000a\u0000l\u0000i\u0000z\u0000i\u0000n\u0000g\u0000 \u0000c\u0000u\u0000r\u0000v\u0000e\u0000 \u0000l\u0000i\u0000b\u0000r\u0000a\u0000r\u0000y\u0000 \u0000.\u0000.\u0000.\u0000 \u0000", "òf¿~“^\u001dRËY\u0016S-N.\u0000.\u0000.\u0000", "á¬ Á\u001cÁà¬|¹ \u0000\bÍ0®TÖiÕÈ²ä².\u0000.\u0000.\u0000"], ["I\u0000n\u0000i\u0000t\u0000i\u0000a\u0000l\u0000i\u0000z\u0000i\u0000n\u0000g\u0000 \u0000s\u0000t\u0000e\u0000p\u0000 \u0000s\u0000e\u0000t\u0000u\u0000p\u0000 \u0000.\u0000.\u0000.\u0000 \u0000", "ek¤š\u001dRËY\u0016S-N.\u0000.\u0000.\u0000", "mÕ©ºÇÌ¸|¹ \u0000\bÍ0®TÖiÕÈ²ä².\u0000.\u0000.\u0000"], ["I\u0000n\u0000i\u0000t\u0000i\u0000a\u0000l\u0000i\u0000z\u0000i\u0000n\u0000g\u0000 \u0000a\u0000d\u0000d\u0000 \u0000s\u0000t\u0000e\u0000p\u0000 \u0000.\u0000.\u0000.\u0000 \u0000", "y˜îv\u001dRËY\u0016S-N.\u0000.\u0000.\u0000", "mÕ©ºÍ\u0000¬ÇÌ¸|¹ \u0000\u0001È¬ÇiÕÈ²ä².\u0000.\u0000.\u0000"], ["I\u0000n\u0000i\u0000t\u0000i\u0000a\u0000l\u0000i\u0000z\u0000i\u0000n\u0000g\u0000 \u0000t\u0000a\u0000s\u0000k\u0000 \u0000s\u0000e\u0000q\u0000u\u0000e\u0000n\u0000c\u0000e\u0000 \u0000.\u0000.\u0000.\u0000", "^\u0017R\u001dRËY\u0016S-N.\u0000.\u0000.\u0000", "ü¬\u001cÈ,¸DÇ \u0000\bÍ0®TÖiÕÈ²ä².\u0000.\u0000.\u0000"], ["I\u0000n\u0000i\u0000t\u0000i\u0000a\u0000l\u0000i\u0000z\u0000i\u0000n\u0000g\u0000 \u0000v\u0000i\u0000r\u0000t\u0000u\u0000a\u0000l\u0000 \u0000d\u0000a\u0000t\u0000a\u0000 \u0000.\u0000.\u0000.\u0000", "—zãS\u001dRËY\u0016S-N.\u0000.\u0000.\u0000", "\u0000¬ÁÀ=Ì8»ÇÌ¸|¹ \u0000\u0001È¬ÇiÕÈ²ä².\u0000.\u0000.\u0000"], ["I\u0000n\u0000i\u0000t\u0000i\u0000a\u0000l\u0000i\u0000z\u0000i\u0000n\u0000g\u0000 \u0000O\u0000p\u0000e\u0000r\u0000a\u0000t\u0000o\u0000r\u0000 \u0000.\u0000.\u0000.\u0000 \u0000", "Íd\\O\u001dRËY\u0016S-N.\u0000.\u0000.\u0000", "äÂÜÂ\u0004¬Ä³l­|¹ \u0000\bÍ0®TÖiÕÈ²ä².\u0000.\u0000.\u0000"], ["L\u0000o\u0000a\u0000d\u0000i\u0000n\u0000g\u0000 \u0000m\u0000a\u0000i\u0000n\u0000 \u0000w\u0000i\u0000n\u0000d\u0000o\u0000w\u0000 \u0000.\u0000.\u0000.\u0000", ";N—zãS\u001dRËY\u0016S-N.\u0000.\u0000.\u0000", "üÈ\u0004Õ\\¸ø­Œ·DÇ \u0000\u0001È¬ÇXÕà¬ˆÇµÂÈ²ä².\u0000.\u0000.\u0000"], ["L\u0000o\u0000a\u0000d\u0000i\u0000n\u0000g\u0000 \u0000m\u0000a\u0000i\u0000n\u0000 \u0000w\u0000i\u0000n\u0000d\u0000o\u0000w\u0000 \u0000.\u0000 \u0000.\u0000", ";N—zãS\u001dRËY\u0016S-N.\u0000 \u0000.\u0000", "üÈ\u0004Õ\\¸ø­Œ·DÇ \u0000\u0001È¬ÇXÕà¬ˆÇµÂÈ²ä².\u0000 \u0000.\u0000"], ["L\u0000o\u0000a\u0000d\u0000i\u0000n\u0000g\u0000 \u0000m\u0000a\u0000i\u0000n\u0000 \u0000w\u0000i\u0000n\u0000d\u0000o\u0000w\u0000 \u0000.\u0000.\u0000 \u0000", ";N—zãS\u001dRËY\u0016S-N.\u0000.\u0000 \u0000", "üÈ\u0004Õ\\¸ø­Œ·DÇ \u0000\u0001È¬ÇXÕà¬ˆÇµÂÈ²ä².\u0000.\u0000 \u0000"], ["V\u0000e\u0000r\u0000s\u0000i\u0000o\u0000n\u0000", "Hr,g", "\u001c¬\u0015Èˆ¼8Ö"], ["H\u0000t\u0000t\u0000p\u0000:\u0000/\u0000/\u0000w\u0000w\u0000w\u0000.\u0000c\u0000r\u0000y\u0000s\u0000o\u0000u\u0000n\u0000d\u0000.\u0000c\u0000o\u0000m\u0000", "lQøSQ@W \u0000:\u0000 \u0000H\u0000t\u0000t\u0000p\u0000:\u0000/\u0000/\u0000w\u0000w\u0000w\u0000.\u0000c\u0000r\u0000y\u0000s\u0000o\u0000u\u0000n\u0000d\u0000.\u0000c\u0000o\u0000m\u0000", "m­\u0000¬ü¬YÕÐÆ \u0000\u0018ÂYÕðÅl­ŒÁ"], ["C\u0000o\u0000p\u0000y\u0000r\u0000i\u0000g\u0000h\u0000t\u0000(\u0000C\u0000)\u0000 \u00002\u00000\u00000\u00009\u0000-\u00002\u00000\u00001\u00004\u0000 \u0000C\u0000R\u0000Y\u0000 \u0000S\u0000o\u0000u\u0000n\u0000d\u0000 \u0000C\u0000o\u0000.\u0000,\u0000 \u0000L\u0000t\u0000d\u0000.\u0000 \u0000A\u0000l\u0000l\u0000 \u0000r\u0000i\u0000g\u0000h\u0000t\u0000s\u0000 \u0000r\u0000e\u0000s\u0000e\u0000r\u0000v\u0000e\u0000d\u0000.\u0000", "HrCg@b\tg(\u0000C\u0000)\u0000 \u00002\u00000\u00000\u00009\u0000-\u00002\u00000\u00001\u00004\u0000 \u0000mgÞ]FQNS5uP[\tgP–lQøS(\u0000\tTØš5uðX)\u0000 \u0000ÝOYu@b\tgCg)R.\u0000", "\u001cÈ‘Ç \u0000:\u0000 \u0000üÈ´Ì1\u00000\u00003\u0000(\u00002\u00000\u00001\u00004\u0000)\u0000D± \u00008\u0000ÔÆ"]]
      # "13"
      n9 = Index Array(array=w29, index (row)=w28) -> (element=w30:string[])  [unwired: 1 in]
      n10 = for {
        tunnel: w30 -> [w34] mode=indexing
        tunnel: [w33] -> w27 mode=indexing
        n11 = global read "CRYMainGlobal.vi" "Full Verion Number Unicode"() -> (w32:string)
        n12 = Concatenate Strings(w34, " \u0000" ("message"), w32) -> (w33:string)
      }
      n13 = Replace Array Subset(array=w29, new element=w27, index (row)=w28) -> (w26:string[][])  [unwired: 1 in]
    }
    frame "About" {
    }
    frame "Main Toolbar" {
      w38 = string[][] [["A\u0000d\u0000d\u0000 \u0000S\u0000t\u0000e\u0000p\u0000", "y˜îvûm R", "mÕ©º”Í\u0000¬"], ["S\u0000t\u0000o\u0000p\u0000", "\\Pbk", "\u0015ÈÀÉ"], ["C\u0000o\u0000n\u0000t\u0000.\u0000", "ç~í~", "Ä¬Á"], ["S\u0000t\u0000o\u0000p\u0000", "\\Pbk", "\u0015ÈÀÉ"], ["R\u0000e\u0000d\u0000o\u0000", "͑\rY", "à¬hÎ"], ["T\u0000i\u0000m\u0000e\u0000", "öeô•", "ÜÂ\u0004¬"], ["P\u0000r\u0000o\u0000j\u0000e\u0000c\u0000t\u0000", "y˜îv¡{\u0006t", "ü¬\u001cÈ,¸"], ["C\u0000u\u0000r\u0000v\u0000e\u0000s\u0000 \u0000L\u0000i\u0000b\u0000r\u0000a\u0000r\u0000y\u0000", "òf¿~“^", "á¬ Á\u001cÁà¬"], ["V\u0000a\u0000l\u0000u\u0000e\u0000 \u0000L\u0000i\u0000b\u0000r\u0000a\u0000r\u0000y\u0000", "pe<P“^", "è²\u001cÂ\u0012¬\u001cÁà¬"], ["R\u0000e\u0000s\u0000u\u0000l\u0000t\u0000 \u0000L\u0000i\u0000b\u0000r\u0000a\u0000r\u0000y\u0000", "Ó~œg“^", "°¬ü¬\u0012¬\u001cÁà¬"], ["W\u0000a\u0000v\u0000e\u0000 \u0000L\u0000i\u0000b\u0000r\u0000a\u0000r\u0000y\u0000", "öeßWâl“^", "ÜÂ\u0004¬\fÓ\u0015Ö\u001cÁà¬"], ["S\u0000t\u0000e\u0000p\u0000 \u0000S\u0000e\u0000t\u0000u\u0000p\u0000", "yîv\u0016", "mÕ©º¸ÓÑÉ"], ["D\u0000a\u0000t\u0000a\u0000 \u0000V\u0000i\u0000e\u0000w\u0000", "°eú^þVhˆ", "ÇÌ¸ô¼0®"], ["D\u0000o\u0000c\u0000u\u0000m\u0000e\u0000n\u0000t\u0000", "¥bJT", "8»\u001cÁ"], ["S\u0000i\u0000g\u0000n\u0000a\u0000l\u0000 \u0000G\u0000e\u0000n\u0000e\u0000r\u0000a\u0000t\u0000o\u0000r\u0000", "áO÷SÑS\u001fuhV", "àÂ8Ö\u001c¼ÝÀ0®"], ["M\u0000u\u0000l\u0000t\u0000i\u0000m\u0000e\u0000t\u0000e\u0000r\u0000", "\u0007N(uhˆ", "Ì¹¥²!Î\u0015ÈÄ¬0®"], ["O\u0000s\u0000c\u0000i\u0000l\u0000l\u0000o\u0000s\u0000c\u0000o\u0000p\u0000e\u0000", ":yâlhV", "$Æ0Å\\¸¤ÂTÏ\u0004Õ"], ["S\u0000p\u0000e\u0000c\u0000t\u0000r\u0000u\u0000m\u0000 \u0000A\u0000n\u0000a\u0000l\u0000y\u0000z\u0000e\u0000r\u0000", "1\u0006RghV", "¤Â™Ó¸Òt¹tÕ\u001dÁ0®"], ["R\u0000e\u0000a\u0000l\u0000 \u0000T\u0000i\u0000m\u0000e\u0000 \u0000A\u0000n\u0000a\u0000l\u0000y\u0000z\u0000e\u0000r\u0000", "\rP\u000bz\u0006RghV", "%ÆÀÐ\f¾ \u0000äÂÜÂ\u0004¬tÕ\u001dÁ"], ["S\u0000t\u0000a\u0000r\u0000t\u0000", "\u0000_ËY", "ÜÂ‘Ç"], ["L\u0000o\u0000t\u0000:\u0000", "ÁT\rT:\u0000", "ˆÔ…º:\u0000"], ["S\u0000/\u0000N\u0000:\u0000", "^÷S:\u0000", "ˆ¼8Ö:\u0000"], ["T\u0000e\u0000s\u0000t\u0000e\u0000d\u0000:\u0000", "KmՋ:\u0000", "€¬¬À:\u0000"], ["M\u0000a\u0000n\u0000u\u0000a\u0000l\u0000", "(u7b\u0007cWS", "$Á…º\u001cÁ"], ["H\u0000o\u0000m\u0000e\u0000 \u0000p\u0000a\u0000g\u0000e\u0000", "Qu˜", "HÖ˜ÓÀÉ"], ["A\u0000b\u0000o\u0000u\u0000t\u0000 \u0000u\u0000s\u0000", "sQŽN¾|ðX", "\u0004Õ\\¸ø­Œ·ÐÅ \u0000\u0000³XÕìÅ"], ["H\u0000a\u0000r\u0000d\u0000w\u0000a\u0000r\u0000e\u0000", "lxöN", "¥ÇXÎ$Á\u0015È"], ["C\u0000a\u0000l\u0000i\u0000b\u0000r\u0000a\u0000t\u0000i\u0000o\u0000n\u0000", "!hÆQ", "P­\u0000É"], ["C\u0000u\u0000r\u0000v\u0000e\u0000 \u0000L\u0000i\u0000b\u0000r\u0000a\u0000r\u0000y\u0000", "òf¿~“^", "á¬ Á\u001cÁà¬"], ["R\u0000u\u0000n\u0000n\u0000i\u0000n\u0000g\u0000", "ck(WÐL", "äÂ‰Õ\u0011É"]]  # Button Label On
      w39 = string[][] [["A\u0000d\u0000d\u0000 \u0000S\u0000t\u0000e\u0000p\u0000", "y˜îvûm R", "mÕ©º”Í\u0000¬"], ["S\u0000t\u0000a\u0000r\u0000t\u0000", "\u0000_ËY", "ÜÂ‘Ç"], ["C\u0000o\u0000n\u0000t\u0000.\u0000", "ç~í~", "Ä¬Á"], ["L\u0000o\u0000o\u0000p\u0000", "Þí~", "(¸Á"], ["R\u0000e\u0000d\u0000o\u0000", "͑\rY", "à¬hÎ"], ["T\u0000i\u0000m\u0000e\u0000", "öeô•", "ÜÂ\u0004¬"], ["P\u0000r\u0000o\u0000j\u0000e\u0000c\u0000t\u0000", "y˜îv¡{\u0006t", "ü¬\u001cÈ,¸"], ["C\u0000u\u0000r\u0000v\u0000e\u0000s\u0000 \u0000L\u0000i\u0000b\u0000r\u0000a\u0000r\u0000y\u0000", "òf¿~“^", "á¬ Á\u001cÁà¬"], ["V\u0000a\u0000l\u0000u\u0000e\u0000 \u0000L\u0000i\u0000b\u0000r\u0000a\u0000r\u0000y\u0000", "pe<P“^", "è²\u001cÂ\u0012¬\u001cÁà¬"], ["R\u0000e\u0000s\u0000u\u0000l\u0000t\u0000 \u0000L\u0000i\u0000b\u0000r\u0000a\u0000r\u0000y\u0000", "Ó~œg“^", "°¬ü¬\u0012¬\u001cÁà¬"], ["W\u0000a\u0000v\u0000e\u0000 \u0000L\u0000i\u0000b\u0000r\u0000a\u0000r\u0000y\u0000", "öeßWâl“^", "ÜÂ\u0004¬\fÓ\u0015Ö\u001cÁà¬"], ["S\u0000t\u0000e\u0000p\u0000 \u0000S\u0000e\u0000t\u0000u\u0000p\u0000", "yîv\u0016", "mÕ©º¸ÓÑÉ"], ["D\u0000a\u0000t\u0000a\u0000 \u0000V\u0000i\u0000e\u0000w\u0000", "°eú^þVhˆ", "ø­|·\u0004Õ"], ["D\u0000o\u0000c\u0000u\u0000m\u0000e\u0000n\u0000t\u0000", "¥bJT", "8»\u001cÁ¸ÓÑÉ"], ["S\u0000i\u0000g\u0000n\u0000a\u0000l\u0000 \u0000G\u0000e\u0000n\u0000e\u0000r\u0000a\u0000t\u0000o\u0000r\u0000", "áO÷SÑS\u001fuhV", "àÂ8Ö\u001c¼ÝÀ0®"], ["M\u0000u\u0000l\u0000t\u0000i\u0000m\u0000e\u0000t\u0000e\u0000r\u0000", "\u0007N(uhˆ", "Ì¹¥²!Î\u0015ÈÄ¬0®"], ["O\u0000s\u0000c\u0000i\u0000l\u0000l\u0000o\u0000s\u0000c\u0000o\u0000p\u0000e\u0000", ":yâlhV", "$Æ0Å\\¸¤ÂTÏ\u0004Õ"], ["S\u0000p\u0000e\u0000c\u0000t\u0000r\u0000u\u0000m\u0000 \u0000A\u0000n\u0000a\u0000l\u0000y\u0000z\u0000e\u0000r\u0000", "1\u0006RghV", "¤Â™Ó¸Òt¹tÕ\u001dÁ0®"], ["R\u0000e\u0000a\u0000l\u0000 \u0000T\u0000i\u0000m\u0000e\u0000 \u0000A\u0000n\u0000a\u0000l\u0000y\u0000z\u0000e\u0000r\u0000", "\rP\u000bz\u0006RghV", "%ÆÀÐ\f¾ \u0000äÂÜÂ\u0004¬tÕ\u001dÁ"], ["P\u0000a\u0000u\u0000s\u0000e\u0000", "\\Pbk", "\u0015ÈÀÉ"], ["L\u0000o\u0000t\u0000:\u0000", "ÁT\rT:\u0000", "ˆÔ…º:\u0000"], ["S\u0000/\u0000N\u0000:\u0000", "^÷S:\u0000", "ˆ¼8Ö:\u0000"], ["T\u0000e\u0000s\u0000t\u0000e\u0000d\u0000:\u0000", "ñ]Km:\u0000", "€¬¬À:\u0000"], ["M\u0000a\u0000n\u0000u\u0000a\u0000l\u0000", "(u7b\u0007cWS", "$Á…º\u001cÁ"], ["H\u0000o\u0000m\u0000e\u0000 \u0000p\u0000a\u0000g\u0000e\u0000", "Qu˜", "HÖ˜ÓÀÉ"], ["A\u0000b\u0000o\u0000u\u0000t\u0000 \u0000u\u0000s\u0000", "sQŽN¾|ðX", "\u0004Õ\\¸ø­Œ·ÐÅ \u0000\u0000³XÕìÅ"], ["H\u0000a\u0000r\u0000d\u0000w\u0000a\u0000r\u0000e\u0000", "lxöN", "¥ÇXÎ$Á\u0015È"], ["C\u0000a\u0000l\u0000i\u0000b\u0000r\u0000a\u0000t\u0000i\u0000o\u0000n\u0000", "!hÆQ", "P­\u0000É"], ["C\u0000u\u0000r\u0000v\u0000e\u0000 \u0000L\u0000i\u0000b\u0000r\u0000a\u0000r\u0000y\u0000", "òf¿~“^", "á¬ Á\u001cÁà¬"], ["R\u0000u\u0000n\u0000n\u0000i\u0000n\u0000g\u0000", "ck(WÐL", "äÂ‰Õ\u0011É"]]  # Button Label Off
      w40 = string[] ["AddStep", "Start", "Seq Continue", "Continue", "Redo", "Elapsed", "Project", "Curve Lib", "Value Lib", "TF Lib", "Wave Lib", "Step Setup", "Data View", "Document", "SignalGen", "MultiMeter", "Oscillo", "Spectral", "RTA", "Pause", "Lot:", "S/N:", "Tested:", "Manual", "Company Site", "About", "SetSoundCard", "SetCalibration", "Curve Library", "Seq running"]  # Control Name
      w43 = string[][] [["A\u0000d\u0000d\u0000 \u0000S\u0000t\u0000e\u0000p\u0000", "y˜îvûm R", "ü¬\u001cÈmÕ©ºDÇ \u0000”Í\u0000¬iÕÈ²ä²"], ["S\u0000t\u0000a\u0000r\u0000t\u0000", "\u0000_ËY", "ü¬\u001cÈ,¸DÇ \u0000äÂ‰ÕiÕÈ²ä²"], ["R\u0000u\u0000n\u0000 \u0000c\u0000o\u0000n\u0000t\u0000i\u0000n\u0000u\u0000e\u0000", "ç~í~", "ü¬\u001cÈ,¸DÇ \u0000Ä¬Á \u0000äÂÕiÕÈ²ä²"], ["R\u0000u\u0000n\u0000 \u0000L\u0000o\u0000o\u0000p\u0000", "Þí~", "ü¬\u001cÈ,¸DÇ \u0000(¸Á\u0001È<Ç\\¸ \u0000äÂÕiÕÈ²ä²"], ["R\u0000e\u0000d\u0000o\u0000", "͑\rY", "¬¬ÀÖ\u0018Â|¹ \u0000É\u0000¬ÜÂ¤ÐÀÉ \u0000JÅà¬ \u0000ä²ÜÂ \u0000äÂÕiÕÈ²ä²"], ["T\u0000i\u0000m\u0000e\u0000", "öeô•", "äÂ‰ÕÜÂ\u0004¬DÇ \u0000\\ÔÜÂiÕÈ²ä²"], ["P\u0000r\u0000o\u0000j\u0000e\u0000c\u0000t\u0000", "^\u0017R\u0016hV", "ü¬\u001cÈ,¸=Ì8» \u0000ô¼0®"], ["C\u0000u\u0000r\u0000v\u0000e\u0000s\u0000 \u0000L\u0000i\u0000b\u0000r\u0000a\u0000r\u0000y\u0000", "òf¿~“^", "á¬ Á\u001cÁà¬=Ì8» \u0000ô¼0®"], ["V\u0000a\u0000l\u0000u\u0000e\u0000 \u0000L\u0000i\u0000b\u0000r\u0000a\u0000r\u0000y\u0000", "pe<P“^", "è²\u001cÂ\u0012¬\u001cÁà¬=Ì8» \u0000ô¼0®"], ["R\u0000e\u0000s\u0000u\u0000l\u0000t\u0000 \u0000L\u0000i\u0000b\u0000r\u0000a\u0000r\u0000y\u0000", "Ó~œg“^", "°¬ü¬\u0012¬\u001cÁà¬=Ì8» \u0000ô¼0®"], ["W\u0000a\u0000v\u0000e\u0000 \u0000L\u0000i\u0000b\u0000r\u0000a\u0000r\u0000y\u0000", "öeßWâl“^", "ÜÂ\u0004¬\fÓ\u0015Ö\u001cÁà¬=Ì8» \u0000ô¼0®"], ["S\u0000t\u0000e\u0000p\u0000 \u0000S\u0000e\u0000t\u0000u\u0000p\u0000", "yîv\u0016", "mÕ©º¸ÓÑÉ=Ì8» \u0000ô¼0®"], ["D\u0000a\u0000t\u0000a\u0000 \u0000V\u0000i\u0000e\u0000w\u0000", "°eú^þVhˆ", "ÇÌ¸ô¼0®=Ì8» \u0000ô¼0®"], ["D\u0000o\u0000c\u0000u\u0000m\u0000e\u0000n\u0000t\u0000", "¥bJT", "8»\u001cÁ¸ÓÑÉ=Ì8» \u0000ô¼0®"], ["S\u0000i\u0000g\u0000n\u0000a\u0000l\u0000 \u0000G\u0000e\u0000n\u0000e\u0000r\u0000a\u0000t\u0000o\u0000r\u0000", "áO÷SÑS\u001fuhV", "àÂ8Ö\u001c¼ÝÀ0®=Ì8» \u0000ô¼0®"], ["M\u0000u\u0000l\u0000t\u0000i\u0000m\u0000e\u0000t\u0000e\u0000r\u0000", "\u0007N(uhˆ", "Ì¹¥²!Î\u0015ÈÄ¬0®=Ì8» \u0000ô¼0®"], ["O\u0000s\u0000c\u0000i\u0000l\u0000l\u0000o\u0000s\u0000c\u0000o\u0000p\u0000e\u0000", ":yâlhV", "$Æ0Å\\¸¤ÂTÏ\u0004Õ=Ì8» \u0000ô¼0®"], ["S\u0000p\u0000e\u0000c\u0000t\u0000r\u0000u\u0000m\u0000 \u0000A\u0000n\u0000a\u0000l\u0000y\u0000z\u0000e\u0000r\u0000", "1\u0006RghV", "¤Â™Ó¸Òt¹tÕ\u001dÁ=Ì8» \u0000ô¼0®"], ["R\u0000e\u0000a\u0000l\u0000 \u0000T\u0000i\u0000m\u0000e\u0000 \u0000A\u0000n\u0000a\u0000l\u0000y\u0000z\u0000e\u0000r\u0000", "\rP\u000bz\u0006RghV", "%ÆÀÐ\f¾tÕ\u001dÁ=Ì8» \u0000ô¼0®"], ["P\u0000a\u0000u\u0000s\u0000e\u0000", "\\Pbk", "\u0015ÈÀÉ"], ["P\u0000r\u0000o\u0000d\u0000u\u0000c\u0000t\u0000 \u0000N\u0000a\u0000m\u0000e\u0000", "ÁT\rT", "ÁÀˆÔ…º"], ["S\u0000e\u0000r\u0000i\u0000a\u0000l\u0000 \u0000N\u0000u\u0000m\u0000b\u0000e\u0000r\u0000", "^÷S", "Ä¬,¸ˆ¼8Ö"], ["T\u0000e\u0000s\u0000t\u0000e\u0000d\u0000 \u0000c\u0000o\u0000u\u0000n\u0000t\u0000", "KmՋpe", "€¬¬À\u0018Â"], ["U\u0000s\u0000e\u0000r\u0000 \u0000M\u0000a\u0000n\u0000u\u0000a\u0000l\u0000", "(u7b\u0007cWS", "$Á…º\u001cÁ"], ["h\u0000t\u0000t\u0000p\u0000:\u0000/\u0000/\u0000w\u0000w\u0000w\u0000.\u0000c\u0000r\u0000y\u0000s\u0000o\u0000u\u0000n\u0000d\u0000.\u0000c\u0000o\u0000m\u0000", "h\u0000t\u0000t\u0000p\u0000:\u0000/\u0000/\u0000w\u0000w\u0000w\u0000.\u0000c\u0000r\u0000y\u0000s\u0000o\u0000u\u0000n\u0000d\u0000.\u0000c\u0000o\u0000m\u0000", "HÖ˜ÓÀÉ"], ["A\u0000b\u0000o\u0000u\u0000t\u0000 \u0000C\u0000R\u0000Y\u00006\u00001\u00008\u00001\u0000", "sQŽN \u0000C\u0000R\u0000Y\u00006\u00001\u00008\u00001\u0000", "\u0004Õ\\¸ø­Œ·ÐÅ \u0000\u0000³XÕìÅ"], ["S\u0000o\u0000u\u0000n\u0000d\u0000C\u0000a\u0000r\u0000d\u0000", "ðXaS", "¥ÇXÎ$Á\u0015ÈDÇ \u0000ÄÉ‰ÕiÕÈ²ä².\u0000"], ["C\u0000a\u0000l\u0000i\u0000b\u0000r\u0000a\u0000t\u0000i\u0000o\u0000n\u0000", "!hÆQ", "P­\u0000ÉDÇ \u0000ÄÉ‰ÕiÕÈ²ä².\u0000"], ["C\u0000u\u0000r\u0000v\u0000e\u0000 \u0000L\u0000i\u0000b\u0000r\u0000a\u0000r\u0000y\u0000", "òf¿~“^", "á¬ Á\u001cÁà¬"], ["R\u0000u\u0000n\u0000n\u0000i\u0000n\u0000g\u0000", "ck(WÐL", "äÂ‰Õ\u0011É"]]  # Button Tooltip
      # "29"
      # "20"
      # "5"
      n14 = Index Array(array=w38, index (col)=w37) -> (element=w36:string[])  [unwired: 1 in]
      n15 = Index Array(array=w39, index (col)=w37) -> (element=w42:string[])  [unwired: 1 in]
      n16 = Index Array(array=w43, index (col)=w37) -> (element=w41:string[])  [unwired: 1 in]
    }
    frame "Common Toolbar" {
      w46 = string[] []  # Control Name
      w47 = string[][] [["C\u0000l\u0000o\u0000s\u0000e\u0000", "sQí•", "ë²0®"], ["H\u0000i\u0000d\u0000e\u0000 \u0000A\u0000u\u0000t\u0000o\u0000", "ê¨RÏ", "=Ì8»ÇÙ³(Â0®0®"], ["F\u0000i\u0000x\u0000", "úVš[", "=Ì8»à¬\u0015È"]]  # Button Tooltip
      n17 = Index Array(array=w47, index (col)=w45) -> (element=w44:string[])  [unwired: 1 in]
    }
    frame "Project" {
      # "8"
    }
    frame "Project Toolbar" {
      w49 = string[] ["TS Name", "Move Down", "Move Up", "Remove", "Property seq", "Property step", "ConfigureShowOnOff", "Expand/Collapse", "Add Step"]  # Control Name
      w50 = string[][] [["T\u0000a\u0000s\u0000k\u0000 \u0000S\u0000e\u0000q\u0000u\u0000e\u0000n\u0000c\u0000e\u0000s\u0000", "^\u0017R", "ü¬\u001cÈ,¸"], ["M\u0000o\u0000v\u0000e\u0000 \u0000D\u0000o\u0000w\u0000n\u0000", "\u000bNûy", "mÕ©ºDÇ \u0000DÅ˜·\\¸ \u0000tÇÙ³"], ["M\u0000o\u0000v\u0000e\u0000 \u0000U\u0000p\u0000", "\nNûy", "mÕ©ºDÇ \u0000°Æ\\¸ \u0000tÇÙ³"], ["D\u0000e\u0000l\u0000e\u0000t\u0000e\u0000 \u0000I\u0000t\u0000e\u0000m\u0000", " Rd–", "mÕ©º \u0000­À\u001cÈ"], ["T\u0000a\u0000s\u0000k\u0000 \u0000S\u0000e\u0000q\u0000u\u0000e\u0000n\u0000c\u0000e\u0000 \u0000P\u0000r\u0000o\u0000p\u0000e\u0000r\u0000t\u0000y\u0000", "^\u0017RMn", "ü¬\u001cÈ,¸ \u0000Á1Á"], ["S\u0000t\u0000e\u0000p\u0000 \u0000P\u0000r\u0000o\u0000p\u0000e\u0000r\u0000t\u0000y\u0000", "ek¤šM‘n", "mÕ©º \u0000Á1Á"], ["C\u0000o\u0000n\u0000f\u0000i\u0000g\u0000u\u0000r\u0000e\u0000S\u0000h\u0000o\u0000w\u0000O\u0000n\u0000O\u0000f\u0000f\u0000", "Ó~„g>f:y\u0000_/\u0000sQ", "l­1Áô¼0®/\u0000(Â0®0®"], ["E\u0000x\u0000p\u0000a\u0000n\u0000d\u0000/\u0000C\u0000o\u0000l\u0000l\u0000a\u0000p\u0000s\u0000e\u0000", "U\\\u0000_/\u00006eÞV", "¼ÓXÎ0®/\u0000\u0011È0®"], ["A\u0000d\u0000d\u0000 \u0000S\u0000t\u0000e\u0000p\u0000", "ûm R", "ü¬\u001cÈmÕ©º”Í\u0000¬"]]  # Button Tooltip
      n18 = Index Array(array=w50, index (col)=w52) -> (element=w51:string[])  [unwired: 1 in]
    }
    frame "Curves Library" {
      # "13"
      # "12"
      # "11"
      # "10"
    }
    frame "Curves Library Toolbar" {
      n19 = Index Array(array=string[][] [["O\u0000p\u0000e\u0000n\u0000", "Sb\u0000_", "ôÅ0®"], ["S\u0000a\u0000v\u0000e\u0000", "ÝOX[", "ô¼\u0000­"], ["D\u0000e\u0000l\u0000e\u0000t\u0000e\u0000", " Rd–", "ÇÌ¸ÀÉ°Æ0®"], ["P\u0000r\u0000o\u0000t\u0000e\u0000c\u0000t\u0000", "ÝO¤b", "ÇÌ¸ô¼8Ö"], ["A\u0000u\u0000t\u0000o\u0000P\u0000r\u0000o\u0000t\u0000e\u0000c\u0000t\u0000", "ê¨RÝO¤b", "ÇÙ³ÇÌ¸ô¼8Ö"], ["U\u0000n\u0000d\u0000o\u0000A\u0000u\u0000t\u0000o\u0000P\u0000r\u0000o\u0000t\u0000e\u0000c\u0000t\u0000", "ÖSmê¨RÝO¤b", "ÇÙ³ÇÌ¸ô¼8ÖtÕ\u001cÈ"], ["C\u0000o\u0000m\u0000p\u0000l\u0000e\u0000t\u0000e\u0000D\u0000e\u0000l\u0000e\u0000t\u0000e\u0000", " Rd–", "ÇÌ¸ÀÉ°Æ0®"]], index (col)=w54) -> (element=w55:string[])  [unwired: 1 in]
    }
    frame "Add Step" {
    }
    frame "Add Step Toolbar" {
      w60 = string[] ["Refresh", "Remove", "Option"]  # Control Name
      w61 = string[][] [["R\u0000e\u0000f\u0000r\u0000e\u0000s\u0000h\u0000", "7R°e", "ä²ÜÂ}Ç0®"], ["R\u0000e\u0000m\u0000o\u0000v\u0000e\u0000", " Rd–", "­À\u001cÈ"], ["O\u0000p\u0000t\u0000i\u0000o\u0000n\u0000", "\ty", "XÖ½¬$Á\u0015È"]]  # Button Tooltip
      n20 = Index Array(array=w61, index (col)=w59) -> (element=w58:string[])  [unwired: 1 in]
    }
    frame "Step Setup" {
    }
    frame "Step Setup Toolbar", "ViewData Toolbar" {
      w63 = string[][] [["O\u0000p\u0000e\u0000n\u0000", "Sb\u0000_", "mÕ©ºôÅ0®"], ["S\u0000a\u0000v\u0000e\u0000 \u0000A\u0000s\u0000", "æSX[:N", "mÕ©ºDÇ \u0000tÇ„¹DÇ \u0000\u0014¼¸¯´Å \u0000ô¼\u0000­"], ["R\u0000e\u0000v\u0000e\u0000r\u0000t\u0000", "b`\rY", "ÇÌ¸Öõ¼"], ["P\u0000r\u0000o\u0000p\u0000e\u0000r\u0000t\u0000y\u0000", "^\\'`", "ø­|·\u0004ÕÁ1Á"], ["T\u0000i\u0000t\u0000l\u0000e\u0000 \u0000S\u0000h\u0000o\u0000w\u0000 \u0000O\u0000n\u0000/\u0000O\u0000f\u0000f\u0000", "\u0007h˜˜>f:y\u0000_/\u0000sQ", "\\Ô\u001cÈ`·ô¼0®/\u0000(Â0®0®"], ["L\u0000e\u0000g\u0000e\u0000n\u0000d\u0000S\u0000h\u0000o\u0000w\u0000O\u0000n\u0000O\u0000f\u0000f\u0000", "þV‹O>f:y\u0000_/\u0000sQ", "tÇ„¹©º]¸ \u0000\\ÔÜÂ/\u0000(Â0®0®"], ["C\u0000u\u0000r\u0000s\u0000o\u0000r\u0000S\u0000h\u0000o\u0000w\u0000O\u0000n\u0000O\u0000f\u0000f\u0000", "IQ\u0007h>f:y\u0000_/\u0000sQ", " Ç\\Ô=Ì8» \u0000\\ÔÜÂ/\u0000(Â0®0®"], ["P\u0000r\u0000e\u0000v\u0000i\u0000e\u0000w\u0000S\u0000h\u0000o\u0000w\u0000O\u0000n\u0000O\u0000f\u0000f\u0000", "„˜È‰>f:y\u0000_/\u0000sQ", "ø»¬¹ô¼0®=Ì8» \u0000\\ÔÜÂ/\u0000(Â0®0®"], ["A\u0000d\u0000d\u0000 \u0000W\u0000a\u0000v\u0000e\u0000 \u0000G\u0000r\u0000a\u0000p\u0000h\u0000", "ûm Râlb_þV", "ÜÂ\u0004¬\fÓ\u0015Öø­|·\u0004Õ \u0000”Í\u0000¬"], ["A\u0000d\u0000d\u0000 \u0000X\u0000Y\u0000 \u0000G\u0000r\u0000a\u0000p\u0000h\u0000", "ûm RX\u0000Y\u0000þV", "X\u0000Y\u0000ø­|·\u0004Õ \u0000”Í\u0000¬"], ["A\u0000d\u0000d\u0000 \u0000P\u0000o\u0000l\u0000a\u0000r\u0000 \u0000G\u0000r\u0000a\u0000p\u0000h\u0000", "ûm RgPW\u0007hþV", "ù­Ç¬¹\\Ôø­|·\u0004Õ \u0000Í\u0000¬"], ["A\u0000d\u0000d\u0000 \u0000T\u0000a\u0000b\u0000l\u0000e\u0000", "ûm Rhˆ<h", "\\Ô \u0000”Í\u0000¬"], ["A\u0000d\u0000d\u0000 \u0000R\u0000e\u0000s\u0000u\u0000l\u0000t\u0000", "ûm RÓ~œg", "°¬ü¬\u0012¬ \u0000”Í\u0000¬"], ["A\u0000d\u0000d\u0000 \u0000O\u0000c\u0000t\u0000a\u0000v\u0000e\u0000 \u0000G\u0000r\u0000a\u0000p\u0000h\u0000", "ûm R\rP‘˜\u000bzþV", "%ÆÀÐ\f¾ø­|·\u0004Õ \u0000”Í\u0000¬"], ["A\u0000d\u0000d\u0000 \u0000T\u0000e\u0000x\u0000t\u0000", "ûm R‡e,g", "ø¼8» \u0000”Í\u0000¬"], ["A\u0000d\u0000d\u0000 \u0000D\u0000i\u0000g\u0000i\u0000t\u0000a\u0000l\u0000 \u0000G\u0000r\u0000a\u0000p\u0000h\u0000", "ûm RpeW[þV", "\u0018ÂÇàÂ8Öø­|·\u0004Õ \u0000Í\u0000¬"], ["A\u0000d\u0000d\u0000 \u0000P\u0000i\u0000c\u0000t\u0000u\u0000r\u0000e\u0000", "ûm RþVÏP", "ø­¼¹ \u0000”Í\u0000¬"], ["A\u0000d\u0000d\u0000 \u0000I\u0000n\u0000t\u0000e\u0000n\u0000s\u0000i\u0000t\u0000y\u0000 \u0000G\u0000r\u0000a\u0000p\u0000h\u0000", "ûm R‘˜1ŒþV", "\u0000¼Ä³ø­|·\u0004Õ \u0000”Í\u0000¬"], ["X\u0000_\u0000A\u0000u\u0000t\u0000o\u0000s\u0000c\u0000a\u0000l\u0000e\u0000", "X\u0000t \u0000ê¨R/\u0000Kb¨R", "X\u0000Í \u0000ÇÙ³/\u0000\u0018ÂÙ³"], ["Y\u00001\u0000_\u0000A\u0000u\u0000t\u0000o\u0000s\u0000c\u0000a\u0000l\u0000e\u0000", "Y\u00001\u0000t \u0000ê¨R/\u0000Kb¨R", "Y\u00001\u0000Í \u0000ÇÙ³/\u0000\u0018ÂÙ³"], ["Y\u00002\u0000_\u0000A\u0000u\u0000t\u0000o\u0000s\u0000c\u0000a\u0000l\u0000e\u0000", "Y\u00002\u0000t \u0000ê¨R/\u0000Kb¨R", "Y\u00002\u0000Í \u0000ÇÙ³/\u0000\u0018ÂÙ³"], ["A\u0000d\u0000d\u0000 \u0000A\u0000l\u0000i\u0000g\u0000n\u0000e\u0000d\u0000 \u0000W\u0000i\u0000n\u0000d\u0000o\u0000w\u0000", "°eú^ù[PŸ„vþVhˆ", "=Ì8»\u0015È,¸"]]  # Button Tooltip
      w64 = string[] ["Load", "Save As", "Revert", "Property", "TitleShowOnOff", "LegendShowOnOff", "CursorShowOnOff", "PreviewShowOnOff", "Wave", "XY", "Polar", "Table", "Result", "Octave", "Text", "Digital", "Picture", "Intensity", "X_Autoscale", "Y1_Autoscale", "Y2_Autoscale", "Align"]  # Control Name
      n21 = Index Array(array=w63, index (col)=w66) -> (element=w65:string[])  [unwired: 1 in]
    }
    frame "ViewData" {
    }
    frame "Document" {
    }
    frame "Document Toolbar" {
      w71 = string[] ["BtnOpen", "Combo Box", "BtnSave", "BtnPrint", "BtnPage", "BtnImage", "BtnLot", "BtnSN", "BtnDATE"]  # Control Name
      w72 = string[][] [["O\u0000p\u0000e\u0000n\u0000", "Sb\u0000_", "8»\u001cÁôÅ0®"], ["E\u0000x\u0000p\u0000o\u0000r\u0000t\u0000 \u0000F\u0000i\u0000l\u0000e\u0000 \u0000F\u0000o\u0000r\u0000m\u0000a\u0000t\u0000", "úQeöN<h\u000f_", "\fÓ|Çô¼\u0000­\u0015ÖÝÂ"], ["E\u0000x\u0000p\u0000o\u0000r\u0000t\u0000", "úQ", "8»\u001cÁœÍl­"], ["P\u0000r\u0000i\u0000n\u0000t\u0000", "SbpS", "xÇÄÁ"], ["P\u0000a\u0000g\u0000e\u0000 \u0000S\u0000e\u0000t\u0000u\u0000p\u0000", "u˜b—¾‹n", "˜ÓÀÉ$Á\u0015È"], ["I\u0000n\u0000s\u0000e\u0000r\u0000t\u0000 \u0000P\u0000i\u0000c\u0000t\u0000u\u0000r\u0000e\u0000", "ÒceQþVÏP", "ø­¼¹½À…Ç"], ["I\u0000n\u0000s\u0000e\u0000r\u0000t\u0000 \u0000P\u0000r\u0000o\u0000d\u0000u\u0000c\u0000t\u0000 \u0000N\u0000a\u0000m\u0000e\u0000", "ÒceQÁT\rT", "ÁÀˆÔ…º½À…Ç"], ["I\u0000n\u0000s\u0000e\u0000r\u0000t\u0000 \u0000S\u0000N\u0000", "ÒceQ^÷S", "Ä¬,¸ˆ¼8Ö½À…Ç"], ["I\u0000n\u0000s\u0000e\u0000r\u0000t\u0000 \u0000D\u0000a\u0000t\u0000e\u0000/\u0000T\u0000i\u0000m\u0000e\u0000", "ÒceQåe\u001fgöeô•", " °ÇÜÂ\u0004¬½ÀÇ"]]  # Button Tooltip
      n22 = Index Array(array=w72, index (col)=w70) -> (element=w69:string[])  [unwired: 1 in]
    }
    frame "Run Project" {
    }
    frame "WAVE" {
    }
    frame "XY" {
    }
    frame "DIGITAL" {
    }
    frame "OCTAVE" {
    }
    frame "POLAR" {
    }
    frame "TEXT" {
    }
    frame "TABLE" {
    }
    frame "PICTURE" {
    }
    frame "RESULT" {
    }
    frame "INTENSITY" {
    }
    frame "Audio Interface" {
    }
    frame "Calibration" {
      # "4"
    }
    frame "Messages" {
    }
    frame "Stimulus" {
    }
    frame "Analysis" {
    }
    frame "Post Processing" {
    }
    frame "Auto Save" {
    }
    frame "Serial No" {
    }
    frame "Recall" {
    }
    frame "Signal Generator" {
    }
    frame "Multimeter" {
    }
    frame "Oscilloscope-FFT" {
    }
    frame "RTA" {
    }
    frame "Operator Configure" {
    }
    frame "CRY6181 One" {
    }
    frame Default {
    }
  }
  "Control Label On" <- w4
  "Control Name" <- w9
  "Control Label Off" <- w5
  n23 = Index Array(array=w13, index (row)="No", index (col)=w2) -> (element=w10:string)
  "Unicode String" <- w10
  n24 = case shown="\"Chinese traditional\"" w3 {
    tunnel: [w100 w101 w102 w103] -> w7
    frame "English", Default {
      w100 = u32 0 items=["System default"=0, "Latin-1"=1252, "Japanese"=932, "Korean"=947, "Chinese simplified"=936, "Chinese traditional"=950, "Central Europe"=1250, "Cyrillic"=1251, "Greek"=1253, "Turkish"=1254, "Hebrew"=1255, "Arabic"=1256, "Baltic"=1257, "Thai"=874, "Vietnamese"=783, "UTF8"=65001, "UTF-7"=65000] ("Code Page")
    }
    frame "Chinese traditional" {
      w101 = u32 950 items=["System default"=0, "Latin-1"=1252, "Japanese"=932, "Korean"=947, "Chinese simplified"=936, "Chinese traditional"=950, "Central Europe"=1250, "Cyrillic"=1251, "Greek"=1253, "Turkish"=1254, "Hebrew"=1255, "Arabic"=1256, "Baltic"=1257, "Thai"=874, "Vietnamese"=783, "UTF8"=65001, "UTF-7"=65000] ("Code Page")
    }
    frame "Chinese" {
      w102 = u32 936 items=["System default"=0, "Latin-1"=1252, "Japanese"=932, "Korean"=947, "Chinese simplified"=936, "Chinese traditional"=950, "Central Europe"=1250, "Cyrillic"=1251, "Greek"=1253, "Turkish"=1254, "Hebrew"=1255, "Arabic"=1256, "Baltic"=1257, "Thai"=874, "Vietnamese"=783, "UTF8"=65001, "UTF-7"=65000] ("Code Page")
    }
    frame "Korean" {
      w103 = u32 949 items=["System default"=0, "Latin-1"=1252, "Japanese"=932, "Korean"=949, "Chinese simplified"=936, "Chinese traditional"=950, "Central Europe"=1250, "Cyrillic"=1251, "Greek"=1253, "Turkish"=1254, "Hebrew"=1255, "Arabic"=1256, "Baltic"=1257, "Thai"=874, "Vietnamese"=783, "UTF8"=65001, "UTF-7"=65000] ("Code Page")
    }
  }
  n25 = for {
    tunnel: w8 -> [w105] mode=indexing
    tunnel: w7 -> [w106]
    tunnel: [w104] -> w6 mode=indexing
    n26 = call "CRYConvert Unicode to Multibyte.vi"("Code Page"=w106, "Unicode String"=w105) -> ("Multibyte string"=w104:string)  [unwired: 8 in, 1 out]
  }
  "Tip Strip" <- w6
  n27 = call "CRYConvert Unicode to Multibyte.vi"("Code Page"=w7, "Unicode String"=w10) -> ("Multibyte string"=→"Multibyte String":string)  [unwired: 8 in, 1 out]
